vi "Test.vi"() -> ()   [LabVIEW 2021]
uses:
  Commander/Commander.lvclass
  C:/Program Files (x86)/Hyper State Machine Framework/SSW_Hyper_State_Machine.lvlibp/State_Machine_Class/Main_State_Machine/Hyper_State_Machine.lvclass
  Common_State/Common_State.lvclass
  Image_Acquisition/Image_Acquisition.lvclass
  Motion_Control/Motion_Control.lvclass
  Data_Logging/Data_Logging.lvclass
  DIO/DIO.lvclass
  C:/Program Files (x86)/Hyper State Machine Framework/SSW_Hyper_State_Machine.lvlibp/State_Machine_Class/State_Machine_Module.llb/State Machine.ctl
  C:/Program Files (x86)/Hyper State Machine Framework/SSW_Hyper_State_Machine.lvlibp/State_Machine_Class/State_Machine_Module.llb/Lock_Unlock.ctl
  C:/Program Files (x86)/Hyper State Machine Framework/SSW_Hyper_State_Machine.lvlibp/State_Machine_Class/State_Machine_Module.llb/Iterval.ctl
  C:/Program Files (x86)/Hyper State Machine Framework/SSW_Hyper_State_Machine.lvlibp/State_Machine_Class/State_Machine_Module.llb/Time_Out.ctl
  <vilib>/numeric/Random Number (Range) DBL.vi
  <vilib>/Utility/High Resolution Relative Seconds.vi
  C:/Program Files (x86)/Hyper State Machine Framework/SSW_Hyper_State_Machine.lvlibp
panel:
  out "Activate":bool
  out "Lamp":bool
  out "Current_Pos":dbl caption="mm"
  in  "EMO":bool
  out "Product ID":string
  in  "Activate_Code(Blank for 30 min Trial)":string="ROeInPkJ3DxAXwEgzbbW2XA0t1jaS1URlS9jikesQMED6VfU"
  out "Heart_Rate":bool
  out "Heart rate(s)":dbl format="%#_6p"
  out "Execute rate(Hz)":dbl format="%#_6p"
  out "Base Class_Time_Act":bool
  out "Base Class_Elapsed Time(s)":dbl format="%#_6p"
  out "Base Class":bool=TRUE
  out "Base Class_Remaining(s)":dbl format="%#_6p"
  out "Base Class Progress":dbl(slide) scale=0.0..10.0
  in  "Base Class":dbl=10.0 max=1000.0 format="%#_13p"
  out "Base Class":string
  out "Base Class_Active":bool
  in  "Action Manager":T1(ring)
  out "Common":bool=TRUE
  out "Common_State":string
  out "Common_Time_Act":bool
  out "Common_Elapsed Time(s)":dbl format="%#_6p"
  out "Common_State Progress":dbl(slide) scale=0.0..5.0
  in  "Common_State_Interval":dbl=5.0 max=1000.0 format="%#_13p"
  out "Common_State_Active":bool
  out "Common_State_Remaining(s)":dbl format="%#_6p"
  out "Data Logging Progress":dbl(slide) scale=0.0..3.0
  out "DIO Progress":dbl(slide) scale=0.0..0.01
  out "Motion Control Progress":dbl(slide) scale=0.0..0.5
  out "Image Acquisition Progress":dbl(slide) scale=0.0..0.25
  out "Commander Progress":dbl(slide)=-1.0 scale=0.0..1.0
  out "Data_Logging":bool=TRUE
  out "Data Logging":string
  out "Data_Logging_Time_Act":bool
  out "Data_Logging_Elapsed Time(s)":dbl format="%#_6p"
  out "DIO":bool=TRUE
  out "DIO":string
  out "DIO_Time_Act":bool
  out "DIO_Elapsed Time(s)":dbl format="%#_6p"
  out "Motion_Control":bool=TRUE
  out "Motion_Control":string
  out "Motion_Control_Time_Act":bool
  out "Motion_Control_Elapsed Time(s)":dbl format="%#_6p"
  in  "Data Logging":dbl=3.0 max=1000.0 format="%#_13p"
  out "Data Logging_Active":bool
  out "Data Logging_Remaining(s)":dbl format="%#_6p"
  in  "DIO_Interval":dbl=0.01 max=1000.0 format="%#_13p"
  in  "Motion_Control_Interval":dbl=0.5 max=1000.0 format="%#_13p"
  out "Motion Control_Act":bool
  out "DIO_Act":bool
  out "DIO_Remaining(s)":dbl format="%#_6p"
  out "Motion_Control_Remaining(s)":dbl format="%#_6p"
  in  "Image Acquisition_Interval":dbl=0.25 max=1000.0 format="%#_13p"
  in  "Commander_Interval":dbl max=1000.0 format="%#_13p"
  in  "System_Wait_Time":dbl=0.025 format="%#_13p"
  out "Commander_Active":bool
  out "Image Acquisition_Act":bool
  out "Image Acquisition_Remaining(s)":dbl format="%#_6p"
  out "Commander_Remaining(s)":dbl format="%#_6p"
  out "Image Acquisition":bool=TRUE
  out "Image Acquisition":string
  out "Commander":bool=TRUE
  out "Image Acquisition_Time_Act":bool
  out "Image Acquisition_Elapsed Time(s)":dbl format="%#_6p"
  out "Commander":string
  out "State1_Time_Act":bool
  out "Commander_Elapsed Time(s)":dbl format="%#_6p"
  in  "Stop":bool
  # "Note : Each State is Waiting Until Commader State Finished on \"Interval_Delay\" and then Unlock"
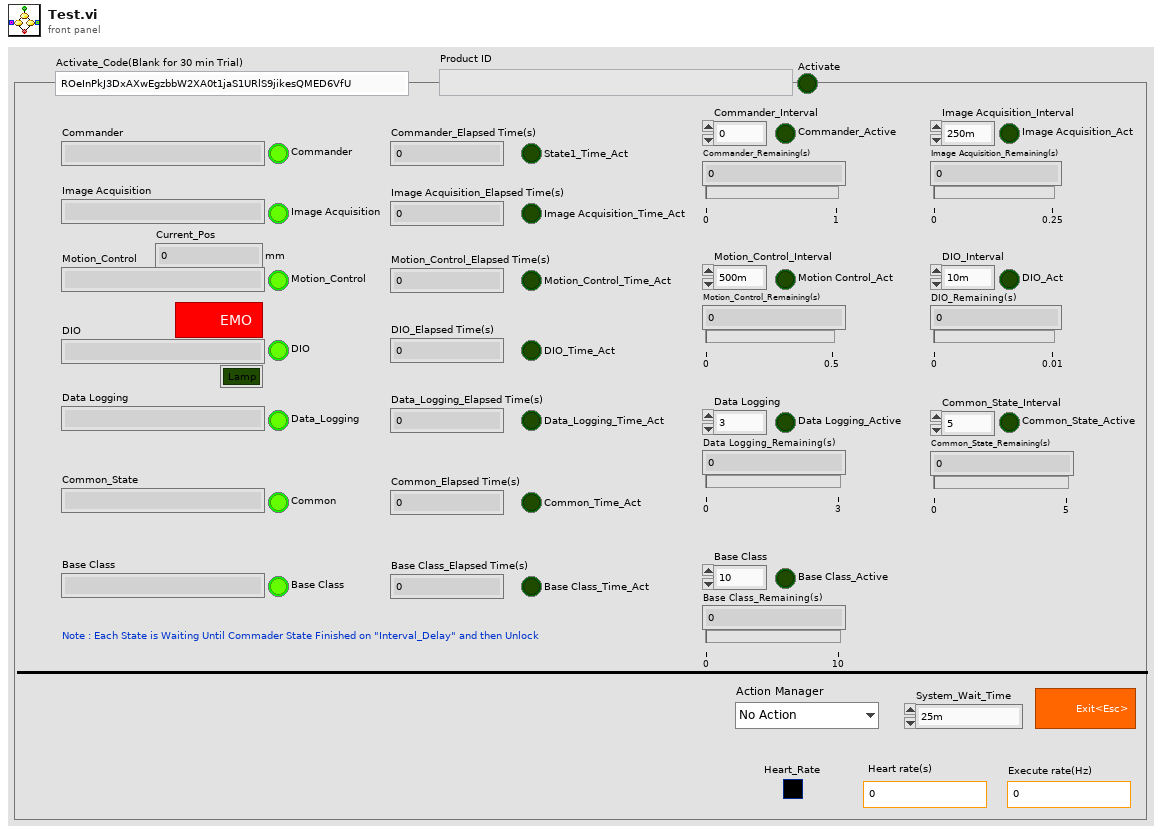
[diagram p1: front panel]
types:
  T1 = enum16{"No Action", "Init", "Lock", "Unlock", "Release"}
  T2 = typedef "SSW_Hyper_State_Machine.lvlibp/State Machine.ctl" = cluster{"Command":string, "Data":variant}
  T3 = typedef "SSW_Hyper_State_Machine.lvlibp/Time_Out.ctl" = cluster{"Enable(True)":bool, "Time Out_State Name":string, "Time Target (1s)":dbl, "Time Out_Reply Message_State":string}
  T4 = typedef "SSW_Hyper_State_Machine.lvlibp/Lock_Unlock.ctl" = cluster{"Action_Mode (Get)":enum16{"Set", "Get"}, "Action_Set (False)":bool, "State_In (Wait)":string}
  T5 = typedef "SSW_Hyper_State_Machine.lvlibp/Iterval.ctl" = cluster{"Delay(s)":dbl, "State (Interval_Delay)":string}
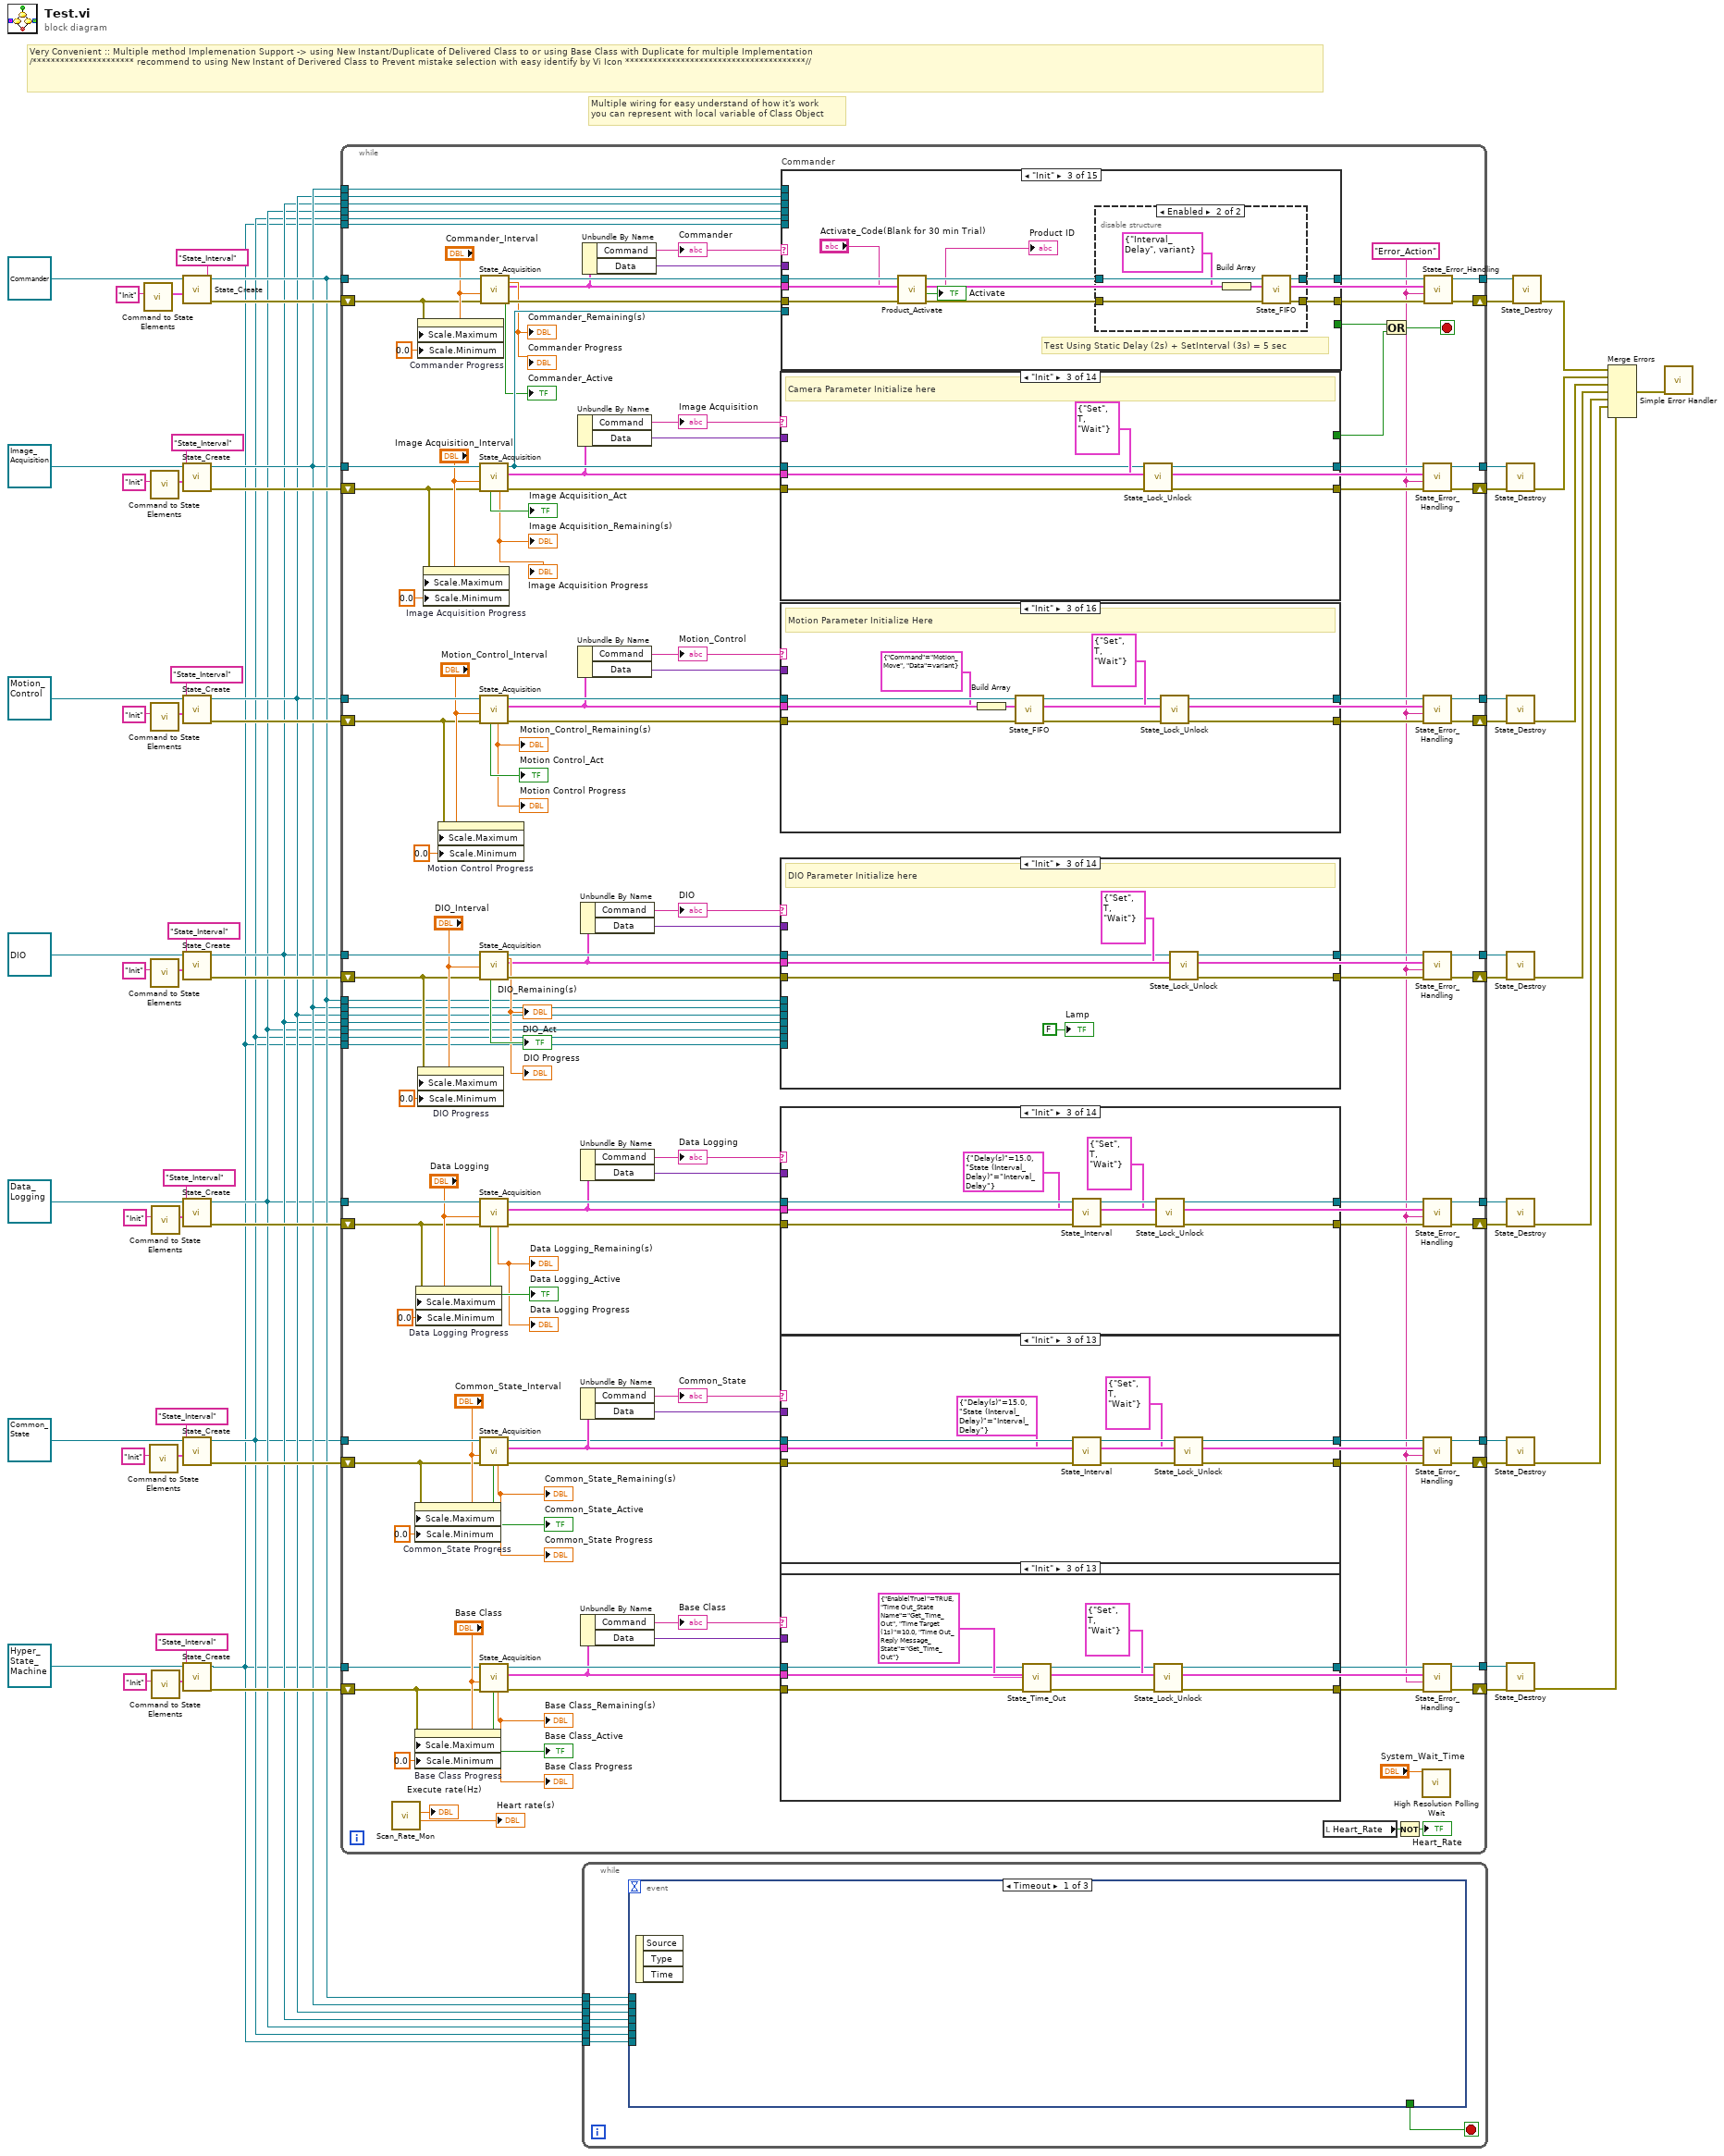
[diagram p0: block diagram]
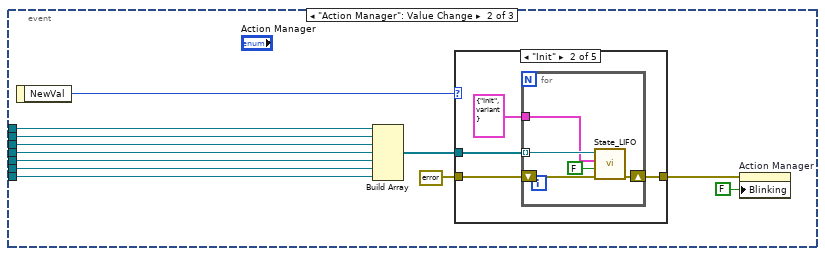
[diagram p2: hidden frame]
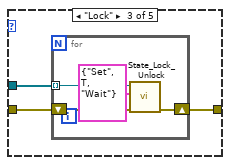
[diagram p4: hidden frame]
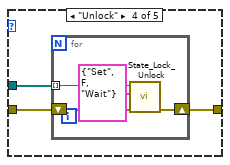
[diagram p5: hidden frame]
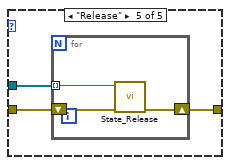
[diagram p6: hidden frame]
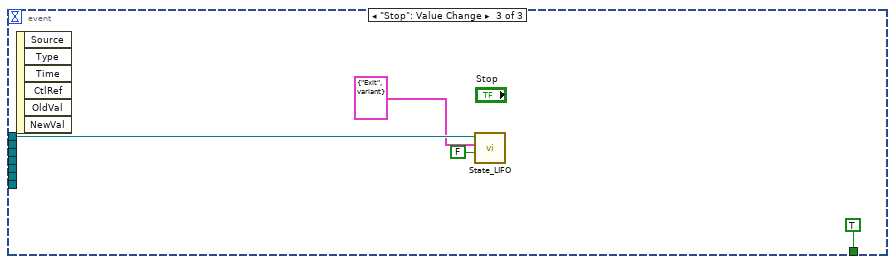
[diagram p7: hidden frame]
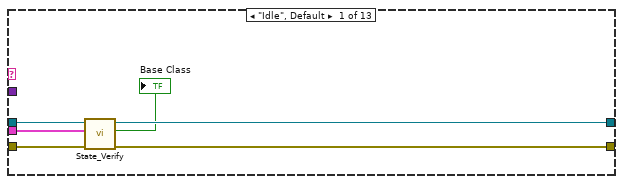
[diagram p8: hidden frame]
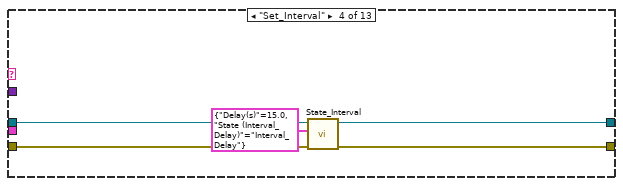
[diagram p10: hidden frame]
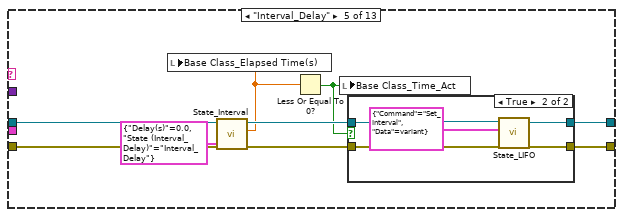
[diagram p11: hidden frame]
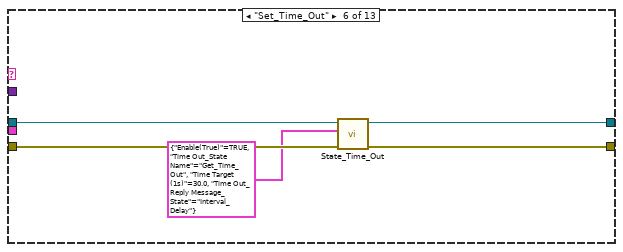
[diagram p13: hidden frame]
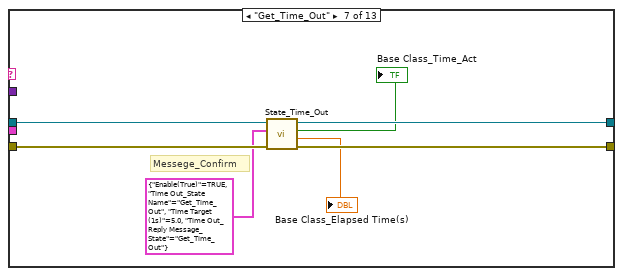
[diagram p14: hidden frame]
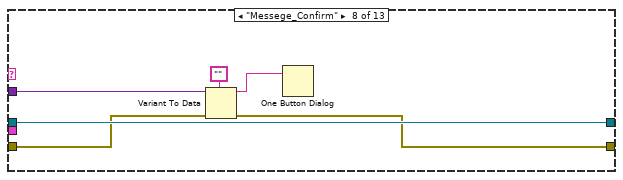
[diagram p15: hidden frame]
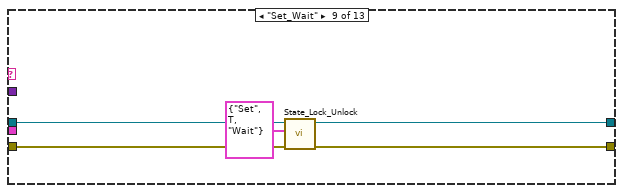
[diagram p16: hidden frame]
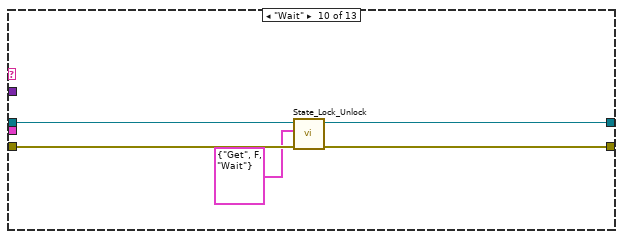
[diagram p17: hidden frame]
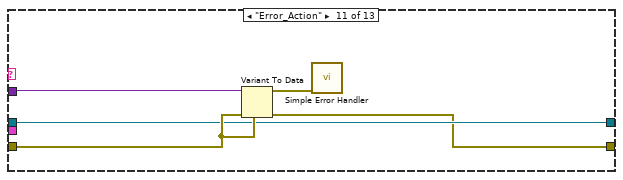
[diagram p18: hidden frame]
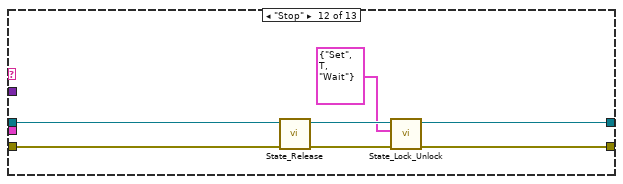
[diagram p19: hidden frame]
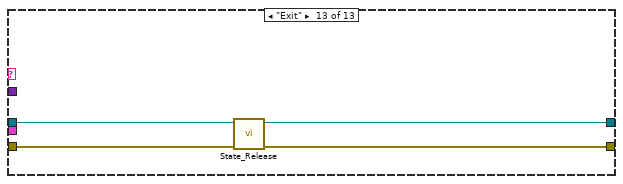
[diagram p20: hidden frame]
diagram:
  # "Multiple wiring for easy understand of how it's work\nyou can represent with local variable of Class Object"
  # "Very Convenient :: Multiple method Implemenation Support -> using New Instant/Duplicate of Delivered Class to or using Base Class with Duplicate for multiple Implementation\n/********************** recommend to using New Instant of Derivered Class to Prevent mistake selection with easy identify by Vi Icon ***************************************//"
  n1 = call "Command to State Elements.vi"("Command"="Init") -> ("Command to State Elements"=w25:T2)  [unwired: 10 in]
  n2 = call "Command to State Elements.vi"("Command"="Init") -> ("Command to State Elements"=w17:T2)  [unwired: 10 in]
  n3 = call "Command to State Elements.vi"("Command"="Init") -> ("Command to State Elements"=w27:T2)  [unwired: 10 in]
  n4 = call "Command to State Elements.vi"("Command"="Init") -> ("Command to State Elements"=w23:T2)  [unwired: 10 in]
  n5 = call "Command to State Elements.vi"("Command"="Init") -> ("Command to State Elements"=w21:T2)  [unwired: 10 in]
  n6 = call "Command to State Elements.vi"("Command"="Init") -> ("Command to State Elements"=w19:T2)  [unwired: 10 in]
  n7 = call "Command to State Elements.vi"("Command"="Init") -> ("Command to State Elements"=w15:T2)  [unwired: 10 in]
  n8 = call-dynamic "State_Create.vi"("Init_State(Option)"=w25, "State_Interval_Name"="State_Interval" ("Core_Interval_Name(State_Interval)"), "State_Machine_Class in"=refnum<class "Commander.lvclass"> refnum ("Commander.lvclass")) -> ("error out"=w64:errorcluster, "State_Machine_Class out"=w7:refnum<class "Commander.lvclass">)  [unwired: 6 in, 1 out]
  n9 = call-dynamic "State_Create.vi"("Init_State(Option)"=w27, "State_Interval_Name"="State_Interval" ("Core_Interval_Name(State_Interval)"), "State_Machine_Class in"=refnum<class "Image_Acquisition.lvclass"> refnum ("Image_Acquisition.lvclass")) -> ("error out"=w61:errorcluster, "State_Machine_Class out"=w6:refnum<class "Image_Acquisition.lvclass">)  [unwired: 6 in, 1 out]
  n10 = call-dynamic "State_Create.vi"("Init_State(Option)"=w23, "State_Interval_Name"="State_Interval" ("Core_Interval_Name(State_Interval)"), "State_Machine_Class in"=refnum<class "Motion_Control.lvclass"> refnum ("Motion_Control.lvclass")) -> ("error out"=w49:errorcluster, "State_Machine_Class out"=w5:refnum<class "Motion_Control.lvclass">)  [unwired: 6 in, 1 out]
  n11 = call-dynamic "State_Create.vi"("Init_State(Option)"=w21, "State_Interval_Name"="State_Interval" ("Core_Interval_Name(State_Interval)"), "State_Machine_Class in"=refnum<class "DIO.lvclass"> refnum ("DIO.lvclass")) -> ("error out"=w47:errorcluster, "State_Machine_Class out"=w4:refnum<class "DIO.lvclass">)  [unwired: 6 in, 1 out]
  n12 = call-dynamic "State_Create.vi"("Init_State(Option)"=w19, "State_Interval_Name"="State_Interval" ("Core_Interval_Name(State_Interval)"), "State_Machine_Class in"=refnum<class "Data_Logging.lvclass"> refnum ("Data_Logging.lvclass")) -> ("error out"=w43:errorcluster, "State_Machine_Class out"=w3:refnum<class "Data_Logging.lvclass">)  [unwired: 6 in, 1 out]
  n13 = call-dynamic "State_Create.vi"("Init_State(Option)"=w17, "State_Interval_Name"="State_Interval" ("Core_Interval_Name(State_Interval)"), "State_Machine_Class in"=refnum<class "Common_State.lvclass"> refnum ("Common_State.lvclass")) -> ("error out"=w38:errorcluster, "State_Machine_Class out"=w2:refnum<class "Common_State.lvclass">)  [unwired: 6 in, 1 out]
  n14 = call-dynamic "State_Create.vi"("Init_State(Option)"=w15, "State_Interval_Name"="State_Interval" ("Core_Interval_Name(State_Interval)"), "State_Machine_Class in"=refnum<class "Hyper_State_Machine.lvclass"> refnum ("SSW_Hyper_State_Machine.lvlibp:Hyper_State_Machine.lvclass")) -> ("error out"=w32:errorcluster, "State_Machine_Class out"=w1:refnum<class "Hyper_State_Machine.lvclass">)  [unwired: 6 in, 1 out]
  n15 = while {
    tunnel: w7 -> [w176]
    shift-right: [w185] -> w63
    shift-left: w64 -> [w84]
    tunnel: [w184] -> w62
    tunnel: w6 -> [w180]
    tunnel: [w179] -> w60
    shift-right: [w178] -> w59
    shift-left: w61 -> [w83]
    tunnel: [w154] -> w51
    tunnel: [w153] -> w50
    tunnel: w5 -> [w152]
    tunnel: w4 -> [w151]
    tunnel: w3 -> [w150]
    shift-right: [w149] -> w48
    shift-left: w49 -> [w82]
    tunnel: [w147] -> w45
    shift-right: [w148] -> w46
    shift-left: w47 -> [w81]
    shift-right: [w146] -> w44
    shift-left: w43 -> [w80]
    tunnel: w2 -> [w125]
    tunnel: [w124] -> w37
    shift-right: [w123] -> w36
    shift-left: w38 -> [w79]
    shift-right: [w93] -> w31
    shift-left: w32 -> [w78]
    tunnel: w1 -> [w97]
    tunnel: [w92] -> w30
    tunnel: w6 -> [w77]
    tunnel: w5 -> [w76]
    tunnel: w4 -> [w75]
    tunnel: w3 -> [w74]
    tunnel: w2 -> [w73]
    tunnel: w1 -> [w72]
    tunnel: w7 -> [w71]
    tunnel: w6 -> [w70]
    tunnel: w5 -> [w69]
    tunnel: w4 -> [w68]
    tunnel: w3 -> [w67]
    tunnel: w2 -> [w66]
    tunnel: w1 -> [w65]
    stop <- w175 stop-if-true
    w91 = "Error_Action" ("State_Error_Handling")
    n16 = call "Scan_Rate_Mon.vi"() -> ("Heart rate(s)"=→"Heart rate(s)":dbl, "Execute rate(Hz)"=→"Execute rate(Hz)":dbl)
    n17 = property on="Common_State Progress" class="Slide (strict)"(error in=w79, "Scale.Maximum"="Common_State_Interval", "Scale.Minimum"=0.0 ("Scale.Range:Minimum")) -> ()  [unwired: 1 in, 2 out]
    n18 = property on="Base Class Progress" class="Slide (strict)"(error in=w78, "Scale.Maximum"="Base Class", "Scale.Minimum"=0.0 ("Scale.Range:Minimum")) -> ()  [unwired: 1 in, 2 out]
    n19 = property on="Data Logging Progress" class="Slide (strict)"(error in=w80, "Scale.Maximum"="Data Logging", "Scale.Minimum"=0.0 ("Scale.Range:Minimum")) -> ()  [unwired: 1 in, 2 out]
    n20 = property on="Commander Progress" class="Slide (strict)"(error in=w84, "Scale.Maximum"="Commander_Interval", "Scale.Minimum"=0.0 ("Scale.Range:Minimum")) -> ()  [unwired: 1 in, 2 out]
    n21 = property on="DIO Progress" class="Slide (strict)"(error in=w81, "Scale.Maximum"="DIO_Interval", "Scale.Minimum"=0.0 ("Scale.Range:Minimum")) -> ()  [unwired: 1 in, 2 out]
    n22 = property on="Image Acquisition Progress" class="Slide (strict)"(error in=w83, "Scale.Maximum"="Image Acquisition_Interval", "Scale.Minimum"=0.0 ("Scale.Range:Minimum")) -> ()  [unwired: 1 in, 2 out]
    n23 = property on="Motion Control Progress" class="Slide (strict)"(error in=w82, "Scale.Maximum"="Motion_Control_Interval", "Scale.Minimum"=0.0 ("Scale.Range:Minimum")) -> ()  [unwired: 1 in, 2 out]
    n24 = call-dynamic "State_Acquisition.vi"("error in (no error)"=w83, "State_Interval_Time(s)"="Image Acquisition_Interval", "Main_Machine_State_Class in"=w180) -> ("error out"=w183:errorcluster, "State"=w110:T2, "Main_Machine_State_Class out"=w177:refnum<class "Image_Acquisition.lvclass">, "Remaining(ms)"=→"Image Acquisition_Remaining(s)" →"Image Acquisition Progress":dbl, "Current_State_Active"=→"Image Acquisition_Act":bool)  [unwired: 2 in, 2 out]
    n25 = call-dynamic "State_Acquisition.vi"("error in (no error)"=w82, "State_Interval_Time(s)"="Motion_Control_Interval", "Main_Machine_State_Class in"=w152) -> ("error out"=w156:errorcluster, "State"=w109:T2, "Main_Machine_State_Class out"=w157:refnum<class "Motion_Control.lvclass">, "Remaining(ms)"=→"Motion_Control_Remaining(s)" →"Motion Control Progress":dbl, "Current_State_Active"=→"Motion Control_Act":bool)  [unwired: 2 in, 2 out]
    n26 = call-dynamic "State_Acquisition.vi"("error in (no error)"=w81, "State_Interval_Time(s)"="DIO_Interval", "Main_Machine_State_Class in"=w151) -> ("error out"=w163:errorcluster, "State"=w108:T2, "Main_Machine_State_Class out"=w164:refnum<class "DIO.lvclass">, "Remaining(ms)"=→"DIO_Remaining(s)" →"DIO Progress":dbl, "Current_State_Active"=→"DIO_Act":bool)  [unwired: 2 in, 2 out]
    n27 = call-dynamic "State_Acquisition.vi"("error in (no error)"=w80, "State_Interval_Time(s)"="Data Logging", "Main_Machine_State_Class in"=w150) -> ("error out"=w165:errorcluster, "State"=w107:T2, "Main_Machine_State_Class out"=w166:refnum<class "Data_Logging.lvclass">, "Remaining(ms)"=→"Data Logging_Remaining(s)" →"Data Logging Progress":dbl, "Current_State_Active"=→"Data Logging_Active":bool)  [unwired: 2 in, 2 out]
    n28 = call-dynamic "State_Acquisition.vi"("error in (no error)"=w79, "State_Interval_Time(s)"="Common_State_Interval", "Main_Machine_State_Class in"=w125) -> ("error out"=w127:errorcluster, "State"=w106:T2, "Main_Machine_State_Class out"=w90:refnum<class "Common_State.lvclass">, "Remaining(ms)"=→"Common_State_Remaining(s)" →"Common_State Progress":dbl, "Current_State_Active"=→"Common_State_Active":bool)  [unwired: 2 in, 2 out]
    n29 = call-dynamic "State_Acquisition.vi"("error in (no error)"=w78, "State_Interval_Time(s)"="Base Class", "Main_Machine_State_Class in"=w97) -> ("error out"=w98:errorcluster, "State"=w95:T2, "Main_Machine_State_Class out"=w99:refnum<class "Hyper_State_Machine.lvclass">, "Remaining(ms)"=→"Base Class_Remaining(s)" →"Base Class Progress":dbl, "Current_State_Active"=→"Base Class_Active":bool)  [unwired: 2 in, 2 out]
    n30 = call-dynamic "State_Acquisition.vi"("error in (no error)"=w84, "State_Interval_Time(s)"="Commander_Interval", "Main_Machine_State_Class in"=w176) -> ("error out"=w187:errorcluster, "State"=w111:T2, "Main_Machine_State_Class out"=w188:refnum<class "Commander.lvclass">, "Remaining(ms)"=→"Commander_Remaining(s)" →"Commander Progress":dbl, "Current_State_Active"=→"Commander_Active":bool)  [unwired: 2 in, 2 out]
    n31 = Unbundle By Name(w110) -> ("Command"=w181:string, "Data"=w182:variant)
    "Image Acquisition" <- w181
    n32 = Unbundle By Name(w109) -> ("Command"=w140:string, "Data"=w169:variant)
    "Motion_Control" <- w140
    n33 = Unbundle By Name(w108) -> ("Command"=w141:string, "Data"=w168:variant)
    "DIO" <- w141
    n34 = Unbundle By Name(w107) -> ("Command"=w142:string, "Data"=w167:variant)
    "Data Logging" <- w142
    n35 = Unbundle By Name(w106) -> ("Command"=w120:string, "Data"=w126:variant)
    "Common_State" <- w120
    n36 = Unbundle By Name(w95) -> ("Command"=w103:string, "Data"=w100:variant)
    "Base Class" <- w103
    n37 = Unbundle By Name(w111) -> ("Command"=w191:string, "Data"=w190:variant)
    "Commander" <- w191
    n38 = case shown="\"Init\"" w181 {
      selector: w181 -> [_ _ _ w666 _ _ _ _ _ _ _ _ _ _]
      tunnel: w182 -> [_ _ _ _ _ _ _ _ w720 _ _ w734 _ _]
      tunnel: w177 -> [w657 w659 w661 w671 w676 w689 w707 w714 w718 w725 w730 w731 w742 w747]
      tunnel: w183 -> [w656 w658 w660 w670 w675 w688 w706 w713 w717 w724 w729 w733 w741 w746]
      tunnel: [w650 w659 w664 w669 w674 w684 w705 w712 w718 w723 w728 w731 w737 w745] -> w171
      tunnel: [w649 w658 w663 w668 w673 w683 w704 w711 w716 w722 w727 w732 w736 w744] -> w170
      tunnel: w110 -> [w655 _ _ _ _ _ _ _ _ _ _ _ _ _]
      tunnel: [_ _ _ _ _ _ _ _ _ _ _ _ _ TRUE] -> w174
      frame "Idle", Default {
        n39 = call-dynamic "State_Verify.vi"("error in (no error)"=w656, "State(Idle)"=w655, "State_Machine_Class in"=w657) -> ("error out"=w652:errorcluster, "Active"=→"Image Acquisition":bool, "State_Machine_Class out"=w653:refnum<class "Image_Acquisition.lvclass">)  [unwired: 6 in]
        n40 = Build Array(T2 {"Command"="Image_Acquisition", "Data"=variant} ("State")) -> (w648:T2[])
        n41 = call-dynamic "State_FIFO.vi"("error in (no error)"=w652, "State Machine[]"=w648, "State_Machine_Class in"=w653) -> ("error out"=w649:errorcluster, "State_Machine_Class out"=w650:refnum<class "Image_Acquisition.lvclass">)  [unwired: 7 in]
      }
      frame "State_Interval" {
      }
      frame "Init" {
        # "Camera Parameter Initialize here"
        n42 = call-dynamic "State_Lock_Unlock.vi"("error in (no error)"=w660, "Parameter"=T4 {"Action_Mode (Get)"=enum."Set", "Action_Set (False)"=TRUE, "State_In (Wait)"="Wait"}, "State_Machine_Class in"=w661) -> ("error out"=w663:errorcluster, "State_Machine_Class out"=w664:refnum<class "Image_Acquisition.lvclass">)  [unwired: 6 in, 1 out]
      }
      frame "Image_Acquisition" {
        (unwired) T5 {"Delay(s)"=5.0, "State (Interval_Delay)"="Image_Acquisition"} ("Parameter")
        # "Simple handling with specify name"
        # "Dynamic handling Name for Waiting Demo"
        # "Image Acquisition Function Here"
        n43 = Bundle By Name(cluster=T5 {"Delay(s)"=5.0, "State (Interval_Delay)"=""} ("Parameter"), "State (Interval_Delay)"=w666) -> (w665:T5)
        n44 = call-dynamic "State_Interval.vi"("error in (no error)"=w670, "Parameter"=w665, "State_Machine_Class in"=w671) -> ("error out"=w668:errorcluster, "State_Machine_Class out"=w669:refnum<class "Image_Acquisition.lvclass">)  [unwired: 6 in, 1 out]
      }
      frame "Set_Interval" {
        n45 = call-dynamic "State_Interval.vi"("error in (no error)"=w675, "Parameter"=T5 {"Delay(s)"=15.0, "State (Interval_Delay)"="Interval_Delay"}, "State_Machine_Class in"=w676) -> ("error out"=w673:errorcluster, "State_Machine_Class out"=w674:refnum<class "Image_Acquisition.lvclass">)  [unwired: 6 in, 1 out]
      }
      frame "Interval_Delay" {
        n46 = call-dynamic "State_Interval.vi"("error in (no error)"=w688, "Parameter"=T5 {"Delay(s)"=0.0, "State (Interval_Delay)"="Interval_Delay"}, "State_Machine_Class in"=w689) -> ("error out"=w685:errorcluster, "Elapsed Time(s)"=w682:dbl, "State_Machine_Class out"=w686:refnum<class "Image_Acquisition.lvclass">)  [unwired: 6 in]
        "Image Acquisition_Elapsed Time(s)" <- w682
        n47 = Build Array(T2 {"Command"="Interval_Delay", "Data"=variant} ("State"), T2 {"Command"="Image_Acquisition", "Data"=variant} ("State")) -> (w678:T2[])
        n48 = Less Or Equal To 0?(x=w682) -> (x <= 0?=w687:bool)
        n49 = Reverse 1D Array(array=w678) -> (reversed array=w677:T2[])
        n50 = case shown="True" w687 {
          tunnel: w686 -> [w691 w696]
          tunnel: w685 -> [w690 w695]
          tunnel: [w691 w694] -> w684
          tunnel: [w690 w693] -> w683
          tunnel: w677 -> [_ w692]
          frame False {
          }
          frame True {
            n51 = for {
              shift-right: [w699] -> w694
              shift-left: w696 -> [w701]
              shift-right: [w698] -> w693
              shift-left: w695 -> [w700]
              tunnel: w692 -> [w697] mode=indexing
              n52 = call-dynamic "State_LIFO.vi"("error in (no error)"=w700, "State Machine"=w697, "State_Machine_Class in"=w701) -> ("error out"=w698:errorcluster, "State_Machine_Class out"=w699:refnum<class "Image_Acquisition.lvclass">)  [unwired: 7 in]
            }
          }
        }
        n53 = local write "Image Acquisition_Time_Act"(w687) -> ()
      }
      frame "Set_Time_Out" {
        n54 = call-dynamic "State_Time_Out.vi"("error in (no error)"=w706, "Parameter"=T3 {"Enable(True)"=TRUE, "Time Out_State Name"="Get_Time_Out", "Time Target (1s)"=30.0, "Time Out_Reply Message_State"="Messege_Confirm"}, "State_Machine_Class in"=w707) -> ("error out"=w704:errorcluster, "Timeout"=w703:bool, "State_Machine_Class out"=w705:refnum<class "Image_Acquisition.lvclass">)  [unwired: 5 in, 1 out]
        n55 = local write "Image Acquisition_Time_Act"(w703) -> ()
      }
      frame "Get_Time_Out" {
        # "Messege_Confirm"
        n56 = call-dynamic "State_Time_Out.vi"("error in (no error)"=w713, "Parameter"=T3 {"Enable(True)"=TRUE, "Time Out_State Name"="Get_Time_Out", "Time Target (1s)"=0.0, "Time Out_Reply Message_State"="Messege_Confirm"}, "State_Machine_Class in"=w714) -> ("error out"=w711:errorcluster, "Remaining Time (s)"=w710:dbl, "Timeout"=→"Image Acquisition_Time_Act":bool, "State_Machine_Class out"=w712:refnum<class "Image_Acquisition.lvclass">)  [unwired: 5 in]
        n57 = local write "Image Acquisition_Elapsed Time(s)"(w710) -> ()
      }
      frame "Messege_Confirm" {
        n58 = Variant To Data(error in=w717, type="", Variant=w720) -> (data=w715:string, error out=w716:errorcluster)
        n59 = One Button Dialog(message=w715) -> ()  [unwired: 1 in, 1 out]
      }
      frame "Set_Wait" {
        n60 = call-dynamic "State_Lock_Unlock.vi"("error in (no error)"=w724, "Parameter"=T4 {"Action_Mode (Get)"=enum."Set", "Action_Set (False)"=TRUE, "State_In (Wait)"="Wait"}, "State_Machine_Class in"=w725) -> ("error out"=w722:errorcluster, "State_Machine_Class out"=w723:refnum<class "Image_Acquisition.lvclass">)  [unwired: 6 in, 1 out]
      }
      frame "Wait" {
        n61 = call-dynamic "State_Lock_Unlock.vi"("error in (no error)"=w729, "Parameter"=T4 {"Action_Mode (Get)"=enum."Get", "Action_Set (False)"=FALSE, "State_In (Wait)"="Wait"}, "State_Machine_Class in"=w730) -> ("error out"=w727:errorcluster, "State_Machine_Class out"=w728:refnum<class "Image_Acquisition.lvclass">)  [unwired: 6 in, 1 out]
      }
      frame "Error_Action" {
        n62 = Variant To Data(error in=w733, type=w733, Variant=w734) -> (data=w735:errorcluster, error out=w732:errorcluster)
        n63 = call <vilib>:"Simple Error Handler.vi"("error in (no error)"=w735) -> ()  [unwired: 4 in, 5 out]
      }
      frame "Stop" {
        n64 = call-dynamic "State_Release.vi"("error in (no error)"=w741, "State_Machine_Class in"=w742) -> ("error out"=w739:errorcluster, "State_Machine_Class out"=w740:refnum<class "Image_Acquisition.lvclass">)  [unwired: 8 in]
        n65 = call-dynamic "State_Lock_Unlock.vi"("error in (no error)"=w739, "Parameter"=T4 {"Action_Mode (Get)"=enum."Set", "Action_Set (False)"=TRUE, "State_In (Wait)"="Wait"}, "State_Machine_Class in"=w740) -> ("error out"=w736:errorcluster, "State_Machine_Class out"=w737:refnum<class "Image_Acquisition.lvclass">)  [unwired: 6 in, 1 out]
      }
      frame "Exit" {
        n66 = call-dynamic "State_Release.vi"("error in (no error)"=w746, "State_Machine_Class in"=w747) -> ("error out"=w744:errorcluster, "State_Machine_Class out"=w745:refnum<class "Image_Acquisition.lvclass">)  [unwired: 8 in]
      }
    }
    n67 = case shown="\"Init\"" w140 {
      tunnel: w169 -> [_ _ _ _ _ _ _ _ _ _ w621 _ _ w634 _ _]
      tunnel: w157 -> [w557 w559 w565 w573 w578 w581 w586 w595 w608 w615 w619 w626 w631 w635 w643 w647]
      tunnel: w156 -> [w556 w558 w563 w572 w577 w580 w585 w594 w607 w614 w618 w625 w630 w633 w642 w646]
      tunnel: [w550 w559 w567 w571 w576 w581 w584 w591 w606 w613 w619 w624 w629 w635 w639 w645] -> w158
      tunnel: [w549 w558 w566 w570 w575 w580 w583 w590 w605 w612 w617 w623 w628 w632 w638 w644] -> w155
      tunnel: w109 -> [w555 _ _ _ _ _ _ _ _ _ _ _ _ _ _ _]
      frame "Idle", Default {
        n68 = call-dynamic "State_Verify.vi"("error in (no error)"=w556, "State(Idle)"=w555, "State_Machine_Class in"=w557) -> ("error out"=w552:errorcluster, "Active"=→"Motion_Control":bool, "State_Machine_Class out"=w553:refnum<class "Motion_Control.lvclass">)  [unwired: 6 in]
        n69 = Build Array(T2 {"Command"="Motion_Move", "Data"=variant} ("State")) -> (w548:T2[])
        n70 = call-dynamic "State_FIFO.vi"("error in (no error)"=w552, "State Machine[]"=w548, "State_Machine_Class in"=w553) -> ("error out"=w549:errorcluster, "State_Machine_Class out"=w550:refnum<class "Motion_Control.lvclass">)  [unwired: 7 in]
      }
      frame "State_Interval" {
        # "Handling Motion I/O or Cirtical Task Here"
      }
      frame "Init" {
        # "Motion Parameter Initialize Here"
        n71 = Build Array(T2 {"Command"="Motion_Move", "Data"=variant} ("State")) -> (w560:T2[])
        n72 = call-dynamic "State_FIFO.vi"("error in (no error)"=w563, "State Machine[]"=w560, "State_Machine_Class in"=w565) -> ("error out"=w562:errorcluster, "State_Machine_Class out"=w564:refnum<class "Motion_Control.lvclass">)  [unwired: 7 in]
        n73 = call-dynamic "State_Lock_Unlock.vi"("error in (no error)"=w562, "Parameter"=T4 {"Action_Mode (Get)"=enum."Set", "Action_Set (False)"=TRUE, "State_In (Wait)"="Wait"}, "State_Machine_Class in"=w564) -> ("error out"=w566:errorcluster, "State_Machine_Class out"=w567:refnum<class "Motion_Control.lvclass">)  [unwired: 6 in, 1 out]
      }
      frame "Motion_Move" {
        # "Motion Move Command here"
        n74 = call-dynamic "State_LIFO.vi"("error in (no error)"=w572, "State Machine"=T2 {"Command"="Motion_Request_Pos", "Data"=variant} ("State"), "State_Machine_Class in"=w573) -> ("error out"=w570:errorcluster, "State_Machine_Class out"=w571:refnum<class "Motion_Control.lvclass">)  [unwired: 7 in]
      }
      frame "Motion_Request_Pos" {
        # "Motion Query Position Command here"
        n75 = call-dynamic "State_LIFO.vi"("error in (no error)"=w577, "State Machine"=T2 {"Command"="Motion_Get_Pos", "Data"=variant} ("State"), "State_Machine_Class in"=w578) -> ("error out"=w575:errorcluster, "State_Machine_Class out"=w576:refnum<class "Motion_Control.lvclass">)  [unwired: 7 in]
      }
      frame "Motion_Get_Pos" {
        # "Motion Move Command here"
        n76 = call-poly <vilib>:"Random Number (Range).vi"() -> ("number"=→"Current_Pos":dbl)  [unwired: 11 in]
      }
      frame "Set_Interval" {
        n77 = call-dynamic "State_Interval.vi"("error in (no error)"=w585, "Parameter"=T5 {"Delay(s)"=15.0, "State (Interval_Delay)"="Interval_Delay"}, "State_Machine_Class in"=w586) -> ("error out"=w583:errorcluster, "State_Machine_Class out"=w584:refnum<class "Motion_Control.lvclass">)  [unwired: 6 in, 1 out]
      }
      frame "Interval_Delay" {
        n78 = call-dynamic "State_Interval.vi"("error in (no error)"=w594, "Parameter"=T5 {"Delay(s)"=0.0, "State (Interval_Delay)"="Interval_Delay"}, "State_Machine_Class in"=w595) -> ("error out"=w592:errorcluster, "Elapsed Time(s)"=w589:dbl, "State_Machine_Class out"=w593:refnum<class "Motion_Control.lvclass">)  [unwired: 6 in]
        n79 = local write "Motion_Control_Elapsed Time(s)"(w589) -> ()
        n80 = Less Or Equal To 0?(x=w589) -> (x <= 0?=w588:bool)
        n81 = local write "Motion_Control_Time_Act"(w588) -> ()
        n82 = case shown="True" w588 {
          tunnel: w593 -> [w597 w603]
          tunnel: w592 -> [w596 w602]
          tunnel: [w597 w601] -> w591
          tunnel: [w596 w600] -> w590
          frame False {
          }
          frame True {
            n83 = call-dynamic "State_LIFO.vi"("error in (no error)"=w602, "State_Interval(Enable)"=FALSE, "State Machine"=T2 {"Command"="Set_Interval", "Data"=variant} ("State"), "State_Machine_Class in"=w603) -> ("error out"=w600:errorcluster, "State_Machine_Class out"=w601:refnum<class "Motion_Control.lvclass">)  [unwired: 6 in]
          }
        }
      }
      frame "Set_Time_Out" {
        n84 = call-dynamic "State_Time_Out.vi"("error in (no error)"=w607, "Parameter"=T3 {"Enable(True)"=TRUE, "Time Out_State Name"="Get_Time_Out", "Time Target (1s)"=30.0, "Time Out_Reply Message_State"="Messege_Confirm"}, "State_Machine_Class in"=w608) -> ("error out"=w605:errorcluster, "State_Machine_Class out"=w606:refnum<class "Motion_Control.lvclass">)  [unwired: 5 in, 2 out]
      }
      frame "Get_Time_Out" {
        # "Messege_Confirm"
        n85 = call-dynamic "State_Time_Out.vi"("error in (no error)"=w614, "Parameter"=T3 {"Enable(True)"=TRUE, "Time Out_State Name"="Get_Time_Out", "Time Target (1s)"=0.0, "Time Out_Reply Message_State"="Messege_Confirm"}, "State_Machine_Class in"=w615) -> ("error out"=w612:errorcluster, "Remaining Time (s)"=→"Motion_Control_Elapsed Time(s)":dbl, "Timeout"=→"Motion_Control_Time_Act":bool, "State_Machine_Class out"=w613:refnum<class "Motion_Control.lvclass">)  [unwired: 5 in]
      }
      frame "Messege_Confirm" {
        n86 = Variant To Data(error in=w618, type="", Variant=w621) -> (data=w616:string, error out=w617:errorcluster)
        n87 = One Button Dialog(message=w616) -> ()  [unwired: 1 in, 1 out]
      }
      frame "Set_Wait" {
        n88 = call-dynamic "State_Lock_Unlock.vi"("error in (no error)"=w625, "Parameter"=T4 {"Action_Mode (Get)"=enum."Set", "Action_Set (False)"=TRUE, "State_In (Wait)"="Wait"}, "State_Machine_Class in"=w626) -> ("error out"=w623:errorcluster, "State_Machine_Class out"=w624:refnum<class "Motion_Control.lvclass">)  [unwired: 6 in, 1 out]
      }
      frame "Wait" {
        n89 = call-dynamic "State_Lock_Unlock.vi"("error in (no error)"=w630, "Parameter"=T4 {"Action_Mode (Get)"=enum."Get", "Action_Set (False)"=FALSE, "State_In (Wait)"="Wait"}, "State_Machine_Class in"=w631) -> ("error out"=w628:errorcluster, "State_Machine_Class out"=w629:refnum<class "Motion_Control.lvclass">)  [unwired: 6 in, 1 out]
      }
      frame "Error_Action" {
        n90 = Variant To Data(error in=w633, type=w633, Variant=w634) -> (data=w636:errorcluster, error out=w632:errorcluster)
        n91 = call <vilib>:"Simple Error Handler.vi"("error in (no error)"=w636) -> ()  [unwired: 4 in, 5 out]
      }
      frame "Stop" {
        n92 = call-dynamic "State_Release.vi"("error in (no error)"=w642, "State_Machine_Class in"=w643) -> ("error out"=w640:errorcluster, "State_Machine_Class out"=w641:refnum<class "Motion_Control.lvclass">)  [unwired: 8 in]
        n93 = call-dynamic "State_Lock_Unlock.vi"("error in (no error)"=w640, "Parameter"=T4 {"Action_Mode (Get)"=enum."Set", "Action_Set (False)"=TRUE, "State_In (Wait)"="Wait"}, "State_Machine_Class in"=w641) -> ("error out"=w638:errorcluster, "State_Machine_Class out"=w639:refnum<class "Motion_Control.lvclass">)  [unwired: 6 in, 1 out]
      }
      frame "Exit" {
        n94 = call-dynamic "State_Release.vi"("error in (no error)"=w646, "State_Machine_Class in"=w647) -> ("error out"=w644:errorcluster, "State_Machine_Class out"=w645:refnum<class "Motion_Control.lvclass">)  [unwired: 8 in]
      }
    }
    n95 = case shown="\"Init\"" w141 {
      tunnel: w168 -> [_ _ _ _ _ _ _ _ w518 _ _ w531 _ _]
      tunnel: w164 -> [w448 w458 w475 w484 w491 w496 w503 w509 w516 w523 w528 w529 w543 w547]
      tunnel: w163 -> [w447 w449 w474 w483 w490 w495 w502 w508 w515 w522 w527 w532 w542 w546]
      tunnel: [w442 w458 w479 w482 w486 w494 w501 w507 w516 w521 w526 w529 w539 w545] -> w162
      tunnel: [w441 w449 w478 w481 w485 w493 w500 w506 w514 w520 w525 w530 w536 w544] -> w161
      tunnel: w108 -> [w446 _ _ _ _ _ _ _ _ _ _ _ _ _]
      tunnel: w71 -> [_ w456 _ _ _ _ _ _ _ _ _ _ _ _]
      tunnel: w70 -> [_ w455 _ _ _ _ _ _ _ _ _ _ _ _]
      tunnel: w69 -> [_ w454 _ _ _ _ _ _ _ _ _ _ _ _]
      tunnel: w68 -> [_ w453 _ _ _ _ _ _ _ _ _ _ _ _]
      tunnel: w67 -> [_ w452 _ _ _ _ _ _ _ _ _ _ _ _]
      tunnel: w66 -> [_ w451 _ _ _ _ _ _ _ _ _ _ _ _]
      tunnel: w65 -> [_ w450 _ _ _ _ _ _ _ _ _ _ _ _]
      frame "Idle", Default {
        # "Able to activate at \"Stae_Interval\""
        n96 = call-dynamic "State_Verify.vi"("error in (no error)"=w447, "State(Idle)"=w446, "State_Machine_Class in"=w448) -> ("error out"=w443:errorcluster, "Active"=→"DIO":bool, "State_Machine_Class out"=w444:refnum<class "DIO.lvclass">)  [unwired: 6 in]
        n97 = Build Array(T2 {"Command"="Lamp_Blinking", "Data"=variant} ("State")) -> (w439:T2[])
        n98 = call-dynamic "State_FIFO.vi"("error in (no error)"=w443, "State Machine[]"=w439, "State_Machine_Class in"=w444) -> ("error out"=w441:errorcluster, "State_Machine_Class out"=w442:refnum<class "DIO.lvclass">)  [unwired: 7 in]
      }
      frame "State_Interval" {
        # "Able to assign to Even to handling"
        # "Simulation of Emergency Signal , Pree to try (Can not Override State Lock if in Active)"
        # "Simulation of Emergency Signal"
        # "Every Cycle Time DIO Get Data Here"
        n99 = case shown="True" "EMO" {
          tunnel: w456 -> [_ w468]
          tunnel: w455 -> [_ w467]
          tunnel: w454 -> [_ w466]
          tunnel: w453 -> [_ w465]
          tunnel: w452 -> [_ w464]
          tunnel: w451 -> [_ w463]
          tunnel: w450 -> [_ w462]
          tunnel: w449 -> [_ w459]
          frame False {
          }
          frame True {
            n100 = Build Array(w468, w467, w466, w465, w464, w463, w462) -> (w461:refnum<class "Hyper_State_Machine.lvclass">[])
            n101 = for {
              tunnel: w461 -> [w473] mode=indexing
              tunnel: T2 {"Command"="Stop", "Data"=variant} ("State") -> [w469]
              shift-right: [w471] -> _
              shift-left: w459 -> [w472]
              n102 = call-dynamic "State_LIFO.vi"("error in (no error)"=w472, "State_Interval(Enable)"=FALSE, "State Machine"=w469, "State_Machine_Class in"=w473) -> ("error out"=w471:errorcluster)  [unwired: 6 in, 1 out]
            }
          }
        }
      }
      frame "Init" {
        # "DIO Parameter Initialize here"
        n103 = call-dynamic "State_Lock_Unlock.vi"("error in (no error)"=w474, "Parameter"=T4 {"Action_Mode (Get)"=enum."Set", "Action_Set (False)"=TRUE, "State_In (Wait)"="Wait"}, "State_Machine_Class in"=w475) -> ("error out"=w478:errorcluster, "State_Machine_Class out"=w479:refnum<class "DIO.lvclass">)  [unwired: 6 in, 1 out]
        "Lamp" <- FALSE ("Lamp")
      }
      frame "Set_Interval" {
        n104 = call-dynamic "State_Interval.vi"("error in (no error)"=w483, "Parameter"=T5 {"Delay(s)"=15.0, "State (Interval_Delay)"="Interval_Delay"}, "State_Machine_Class in"=w484) -> ("error out"=w481:errorcluster, "State_Machine_Class out"=w482:refnum<class "DIO.lvclass">)  [unwired: 6 in, 1 out]
      }
      frame "Interval_Delay" {
        n105 = call-dynamic "State_Interval.vi"("error in (no error)"=w490, "Parameter"=T5 {"Delay(s)"=0.0, "State (Interval_Delay)"="Interval_Delay"}, "State_Machine_Class in"=w491) -> ("error out"=w485:errorcluster, "Elapsed Time(s)"=w489:dbl, "State_Machine_Class out"=w486:refnum<class "DIO.lvclass">)  [unwired: 6 in]
        n106 = local write "DIO_Elapsed Time(s)"(w489) -> ()
        n107 = Less Or Equal To 0?(x=w489) -> (x <= 0?=w488:bool)
        n108 = local write "DIO_Time_Act"(w488) -> ()
      }
      frame "Set_Time_Out" {
        n109 = call-dynamic "State_Time_Out.vi"("error in (no error)"=w495, "Parameter"=T3 {"Enable(True)"=TRUE, "Time Out_State Name"="Get_Time_Out", "Time Target (1s)"=30.0, "Time Out_Reply Message_State"="Messege_Confirm"}, "State_Machine_Class in"=w496) -> ("error out"=w493:errorcluster, "State_Machine_Class out"=w494:refnum<class "DIO.lvclass">)  [unwired: 5 in, 2 out]
      }
      frame "Get_Time_Out" {
        # "Messege_Confirm"
        n110 = call-dynamic "State_Time_Out.vi"("error in (no error)"=w502, "Parameter"=T3 {"Enable(True)"=TRUE, "Time Out_State Name"="Get_Time_Out", "Time Target (1s)"=0.0, "Time Out_Reply Message_State"="Messege_Confirm"}, "State_Machine_Class in"=w503) -> ("error out"=w500:errorcluster, "Remaining Time (s)"=→"DIO_Elapsed Time(s)":dbl, "Timeout"=→"DIO_Time_Act":bool, "State_Machine_Class out"=w501:refnum<class "DIO.lvclass">)  [unwired: 5 in]
      }
      frame "Lamp_Blinking" {
        n111 = call-dynamic "State_Interval.vi"("error in (no error)"=w508, "Parameter"=T5 {"Delay(s)"=0.25, "State (Interval_Delay)"="Lamp_Blinking"}, "State_Machine_Class in"=w509) -> ("error out"=w506:errorcluster, "Elapsed Time(s)"=w504:dbl, "State_Machine_Class out"=w507:refnum<class "DIO.lvclass">)  [unwired: 6 in]
        n112 = Less Or Equal To 0?(x=w504) -> (x <= 0?=w505:bool)
        n113 = case shown="True" w505 {
          frame False {
          }
          frame True {
            n114 = local read "Lamp"() -> (w512:bool)
            n115 = Not(x=w512) -> (.not. x?=w511:bool)
            n116 = local write "Lamp"(w511) -> ()
          }
        }
      }
      frame "Messege_Confirm" {
        n117 = Variant To Data(error in=w515, type="", Variant=w518) -> (data=w513:string, error out=w514:errorcluster)
        n118 = One Button Dialog(message=w513) -> ()  [unwired: 1 in, 1 out]
      }
      frame "Set_Wait" {
        n119 = call-dynamic "State_Lock_Unlock.vi"("error in (no error)"=w522, "Parameter"=T4 {"Action_Mode (Get)"=enum."Set", "Action_Set (False)"=TRUE, "State_In (Wait)"="Wait"}, "State_Machine_Class in"=w523) -> ("error out"=w520:errorcluster, "State_Machine_Class out"=w521:refnum<class "DIO.lvclass">)  [unwired: 6 in, 1 out]
      }
      frame "Wait" {
        n120 = call-dynamic "State_Lock_Unlock.vi"("error in (no error)"=w527, "Parameter"=T4 {"Action_Mode (Get)"=enum."Get", "Action_Set (False)"=FALSE, "State_In (Wait)"="Wait"}, "State_Machine_Class in"=w528) -> ("error out"=w525:errorcluster, "State_Machine_Class out"=w526:refnum<class "DIO.lvclass">)  [unwired: 6 in, 1 out]
      }
      frame "Error_Action" {
        n121 = Variant To Data(error in=w532, type=w532, Variant=w531) -> (data=w533:errorcluster, error out=w530:errorcluster)
        n122 = call <vilib>:"Simple Error Handler.vi"("error in (no error)"=w533) -> ()  [unwired: 4 in, 5 out]
      }
      frame "Stop" {
        n123 = call-dynamic "State_Release.vi"("error in (no error)"=w542, "State_Machine_Class in"=w543) -> ("error out"=w540:errorcluster, "State_Machine_Class out"=w541:refnum<class "DIO.lvclass">)  [unwired: 8 in]
        n124 = call-dynamic "State_Lock_Unlock.vi"("error in (no error)"=w540, "Parameter"=T4 {"Action_Mode (Get)"=enum."Set", "Action_Set (False)"=TRUE, "State_In (Wait)"="Wait"}, "State_Machine_Class in"=w541) -> ("error out"=w537:errorcluster, "State_Machine_Class out"=w539:refnum<class "DIO.lvclass">)  [unwired: 6 in, 1 out]
        n125 = property on="Action Manager" class="Enum (strict)"(error in=w537, "Blinking"=TRUE) -> (error out=w536:errorcluster)  [unwired: 1 in, 1 out]
        n126 = One Button Dialog(message="All State is Locking !\nPlease Unlock With Action Manager to Release . . .") -> ()  [unwired: 1 in, 1 out]
      }
      frame "Exit" {
        n127 = call-dynamic "State_Release.vi"("error in (no error)"=w546, "State_Machine_Class in"=w547) -> ("error out"=w544:errorcluster, "State_Machine_Class out"=w545:refnum<class "DIO.lvclass">)  [unwired: 8 in]
      }
    }
    n128 = case shown="\"Init\"" w142 {
      tunnel: w167 -> [_ _ _ _ _ _ _ _ w412 _ _ w425 _ _]
      tunnel: w166 -> [w360 w362 w370 w372 w377 w386 w399 w406 w410 w417 w422 w424 w434 w438]
      tunnel: w165 -> [w359 w361 w369 w371 w376 w385 w398 w405 w409 w416 w421 w426 w433 w437]
      tunnel: [w357 w362 w366 w372 w375 w382 w397 w404 w410 w415 w420 w424 w429 w436] -> w160
      tunnel: [w356 w361 w365 w371 w374 w381 w396 w403 w408 w414 w419 w423 w428 w435] -> w159
      tunnel: w107 -> [w358 _ _ _ _ _ _ _ _ _ _ _ _ _]
      frame "Idle", Default {
        n129 = call-dynamic "State_Verify.vi"("error in (no error)"=w359, "State(Idle)"=w358, "State_Machine_Class in"=w360) -> ("error out"=w356:errorcluster, "Active"=→"Data_Logging":bool, "State_Machine_Class out"=w357:refnum<class "Data_Logging.lvclass">)  [unwired: 6 in]
      }
      frame "State_Interval" {
        # "Files Monitering or Cirtical Task Handling Here"
      }
      frame "Init" {
        n130 = call-dynamic "State_Interval.vi"("error in (no error)"=w369, "Parameter"=T5 {"Delay(s)"=15.0, "State (Interval_Delay)"="Interval_Delay"}, "State_Machine_Class in"=w370) -> ("error out"=w364:errorcluster, "State_Machine_Class out"=w367:refnum<class "Data_Logging.lvclass">)  [unwired: 6 in, 1 out]
        n131 = call-dynamic "State_Lock_Unlock.vi"("error in (no error)"=w364, "Parameter"=T4 {"Action_Mode (Get)"=enum."Set", "Action_Set (False)"=TRUE, "State_In (Wait)"="Wait"}, "State_Machine_Class in"=w367) -> ("error out"=w365:errorcluster, "State_Machine_Class out"=w366:refnum<class "Data_Logging.lvclass">)  [unwired: 6 in, 1 out]
      }
      frame "Data_Logging" {
        # "Save Data Files Here"
      }
      frame "Set_Interval" {
        n132 = call-dynamic "State_Interval.vi"("error in (no error)"=w376, "Parameter"=T5 {"Delay(s)"=15.0, "State (Interval_Delay)"="Interval_Delay"}, "State_Machine_Class in"=w377) -> ("error out"=w374:errorcluster, "State_Machine_Class out"=w375:refnum<class "Data_Logging.lvclass">)  [unwired: 6 in, 1 out]
      }
      frame "Interval_Delay" {
        n133 = call-dynamic "State_Interval.vi"("error in (no error)"=w385, "Parameter"=T5 {"Delay(s)"=0.0, "State (Interval_Delay)"="Interval_Delay"}, "State_Machine_Class in"=w386) -> ("error out"=w383:errorcluster, "Elapsed Time(s)"=w380:dbl, "State_Machine_Class out"=w384:refnum<class "Data_Logging.lvclass">)  [unwired: 6 in]
        n134 = local write "Data_Logging_Elapsed Time(s)"(w380) -> ()
        n135 = Less Or Equal To 0?(x=w380) -> (x <= 0?=w379:bool)
        n136 = local write "Data_Logging_Time_Act"(w379) -> ()
        n137 = case shown="True" w379 {
          tunnel: w384 -> [w388 w394]
          tunnel: w383 -> [w387 w393]
          tunnel: [w388 w392] -> w382
          tunnel: [w387 w391] -> w381
          frame False {
          }
          frame True {
            n138 = call-dynamic "State_LIFO.vi"("error in (no error)"=w393, "State_Interval(Enable)"=FALSE, "State Machine"=T2 {"Command"="Set_Interval", "Data"=variant} ("State"), "State_Machine_Class in"=w394) -> ("error out"=w391:errorcluster, "State_Machine_Class out"=w392:refnum<class "Data_Logging.lvclass">)  [unwired: 6 in]
          }
        }
      }
      frame "Set_Time_Out" {
        n139 = call-dynamic "State_Time_Out.vi"("error in (no error)"=w398, "Parameter"=T3 {"Enable(True)"=TRUE, "Time Out_State Name"="Get_Time_Out", "Time Target (1s)"=30.0, "Time Out_Reply Message_State"="Interval_Delay"}, "State_Machine_Class in"=w399) -> ("error out"=w396:errorcluster, "State_Machine_Class out"=w397:refnum<class "Data_Logging.lvclass">)  [unwired: 5 in, 2 out]
      }
      frame "Get_Time_Out" {
        # "Messege_Confirm"
        n140 = call-dynamic "State_Time_Out.vi"("error in (no error)"=w405, "Parameter"=T3 {"Enable(True)"=TRUE, "Time Out_State Name"="Get_Time_Out", "Time Target (1s)"=0.0, "Time Out_Reply Message_State"="Messege_Confirm"}, "State_Machine_Class in"=w406) -> ("error out"=w403:errorcluster, "Remaining Time (s)"=→"Data_Logging_Elapsed Time(s)":dbl, "Timeout"=→"Data_Logging_Time_Act":bool, "State_Machine_Class out"=w404:refnum<class "Data_Logging.lvclass">)  [unwired: 5 in]
      }
      frame "Messege_Confirm" {
        n141 = Variant To Data(error in=w409, type="", Variant=w412) -> (data=w407:string, error out=w408:errorcluster)
        n142 = One Button Dialog(message=w407) -> ()  [unwired: 1 in, 1 out]
      }
      frame "Set_Wait" {
        n143 = call-dynamic "State_Lock_Unlock.vi"("error in (no error)"=w416, "Parameter"=T4 {"Action_Mode (Get)"=enum."Set", "Action_Set (False)"=TRUE, "State_In (Wait)"="Wait"}, "State_Machine_Class in"=w417) -> ("error out"=w414:errorcluster, "State_Machine_Class out"=w415:refnum<class "Data_Logging.lvclass">)  [unwired: 6 in, 1 out]
      }
      frame "Wait" {
        n144 = call-dynamic "State_Lock_Unlock.vi"("error in (no error)"=w421, "Parameter"=T4 {"Action_Mode (Get)"=enum."Get", "Action_Set (False)"=TRUE, "State_In (Wait)"="Wait"}, "State_Machine_Class in"=w422) -> ("error out"=w419:errorcluster, "State_Machine_Class out"=w420:refnum<class "Data_Logging.lvclass">)  [unwired: 6 in, 1 out]
      }
      frame "Error_Action" {
        n145 = Variant To Data(error in=w426, type=w426, Variant=w425) -> (data=w427:errorcluster, error out=w423:errorcluster)
        n146 = call <vilib>:"Simple Error Handler.vi"("error in (no error)"=w427) -> ()  [unwired: 4 in, 5 out]
      }
      frame "Stop" {
        n147 = call-dynamic "State_Release.vi"("error in (no error)"=w433, "State_Machine_Class in"=w434) -> ("error out"=w431:errorcluster, "State_Machine_Class out"=w432:refnum<class "Data_Logging.lvclass">)  [unwired: 8 in]
        n148 = call-dynamic "State_Lock_Unlock.vi"("error in (no error)"=w431, "Parameter"=T4 {"Action_Mode (Get)"=enum."Set", "Action_Set (False)"=TRUE, "State_In (Wait)"="Wait"}, "State_Machine_Class in"=w432) -> ("error out"=w428:errorcluster, "State_Machine_Class out"=w429:refnum<class "Data_Logging.lvclass">)  [unwired: 6 in, 1 out]
      }
      frame "Exit" {
        n149 = call-dynamic "State_Release.vi"("error in (no error)"=w437, "State_Machine_Class in"=w438) -> ("error out"=w435:errorcluster, "State_Machine_Class out"=w436:refnum<class "Data_Logging.lvclass">)  [unwired: 8 in]
      }
    }
    n150 = case shown="\"Init\"" w120 {
      tunnel: w126 -> [_ _ _ _ _ _ _ w328 _ _ w342 _ _]
      tunnel: w90 -> [w278 w280 w288 w293 w294 w315 w322 w326 w333 w338 w340 w350 w354]
      tunnel: w127 -> [w277 w279 w287 w292 w302 w314 w321 w325 w332 w337 w341 w349 w353]
      tunnel: [w275 w280 w282 w291 w299 w313 w320 w326 w331 w336 w340 w345 w352] -> w128
      tunnel: [w274 w279 w281 w290 w298 w312 w319 w324 w330 w335 w339 w344 w351] -> w129
      tunnel: w106 -> [w276 _ _ _ _ _ _ _ _ _ _ _ _]
      frame "Idle", Default {
        n151 = call-dynamic "State_Verify.vi"("error in (no error)"=w277, "State(Idle)"=w276, "State_Machine_Class in"=w278) -> ("error out"=w274:errorcluster, "Active"=→"Common":bool, "State_Machine_Class out"=w275:refnum<class "Common_State.lvclass">)  [unwired: 6 in]
      }
      frame "State_Interval" {
        # "Cirtical Task Handling Here"
      }
      frame "Init" {
        n152 = call-dynamic "State_Interval.vi"("error in (no error)"=w287, "Parameter"=T5 {"Delay(s)"=15.0, "State (Interval_Delay)"="Interval_Delay"}, "State_Machine_Class in"=w288) -> ("error out"=w284:errorcluster, "State_Machine_Class out"=w285:refnum<class "Common_State.lvclass">)  [unwired: 6 in, 1 out]
        n153 = call-dynamic "State_Lock_Unlock.vi"("error in (no error)"=w284, "Parameter"=T4 {"Action_Mode (Get)"=enum."Set", "Action_Set (False)"=TRUE, "State_In (Wait)"="Wait"}, "State_Machine_Class in"=w285) -> ("error out"=w281:errorcluster, "State_Machine_Class out"=w282:refnum<class "Common_State.lvclass">)  [unwired: 6 in, 1 out]
      }
      frame "Set_Interval" {
        n154 = call-dynamic "State_Interval.vi"("error in (no error)"=w292, "Parameter"=T5 {"Delay(s)"=15.0, "State (Interval_Delay)"="Interval_Delay"}, "State_Machine_Class in"=w293) -> ("error out"=w290:errorcluster, "State_Machine_Class out"=w291:refnum<class "Common_State.lvclass">)  [unwired: 6 in, 1 out]
      }
      frame "Interval_Delay" {
        n155 = call-dynamic "State_Interval.vi"("error in (no error)"=w302, "Parameter"=T5 {"Delay(s)"=5.0, "State (Interval_Delay)"="Interval_Delay"}, "State_Machine_Class in"=w294) -> ("error out"=w300:errorcluster, "Elapsed Time(s)"=w297:dbl, "State_Machine_Class out"=w301:refnum<class "Common_State.lvclass">)  [unwired: 6 in]
        n156 = local write "Common_Elapsed Time(s)"(w297) -> ()
        n157 = Less Or Equal To 0?(x=w297) -> (x <= 0?=w296:bool)
        n158 = local write "Common_Time_Act"(w296) -> ()
        n159 = case shown="True" w296 {
          tunnel: w301 -> [w304 w310]
          tunnel: w300 -> [w303 w309]
          tunnel: [w304 w308] -> w299
          tunnel: [w303 w307] -> w298
          frame False {
          }
          frame True {
            n160 = call-dynamic "State_LIFO.vi"("error in (no error)"=w309, "State_Interval(Enable)"=FALSE, "State Machine"=T2 {"Command"="Interval_Delay", "Data"=variant} ("State"), "State_Machine_Class in"=w310) -> ("error out"=w307:errorcluster, "State_Machine_Class out"=w308:refnum<class "Common_State.lvclass">)  [unwired: 6 in]
          }
        }
      }
      frame "Set_Time_Out" {
        n161 = call-dynamic "State_Time_Out.vi"("error in (no error)"=w314, "Parameter"=T3 {"Enable(True)"=TRUE, "Time Out_State Name"="Get_Time_Out", "Time Target (1s)"=30.0, "Time Out_Reply Message_State"="Interval_Delay"}, "State_Machine_Class in"=w315) -> ("error out"=w312:errorcluster, "State_Machine_Class out"=w313:refnum<class "Common_State.lvclass">)  [unwired: 5 in, 2 out]
      }
      frame "Get_Time_Out" {
        # "Messege_Confirm"
        # "Messege_Confirm"
        n162 = call-dynamic "State_Time_Out.vi"("error in (no error)"=w321, "Parameter"=T3 {"Enable(True)"=TRUE, "Time Out_State Name"="Get_Time_Out", "Time Target (1s)"=0.0, "Time Out_Reply Message_State"="Set_Interval"}, "State_Machine_Class in"=w322) -> ("error out"=w319:errorcluster, "Remaining Time (s)"=→"Common_Elapsed Time(s)":dbl, "Timeout"=→"Common_Time_Act":bool, "State_Machine_Class out"=w320:refnum<class "Common_State.lvclass">)  [unwired: 5 in]
      }
      frame "Messege_Confirm" {
        n163 = Variant To Data(error in=w325, type="", Variant=w328) -> (data=w323:string, error out=w324:errorcluster)
        n164 = One Button Dialog(message=w323) -> ()  [unwired: 1 in, 1 out]
      }
      frame "Set_Wait" {
        n165 = call-dynamic "State_Lock_Unlock.vi"("error in (no error)"=w332, "Parameter"=T4 {"Action_Mode (Get)"=enum."Set", "Action_Set (False)"=TRUE, "State_In (Wait)"="Wait"}, "State_Machine_Class in"=w333) -> ("error out"=w330:errorcluster, "State_Machine_Class out"=w331:refnum<class "Common_State.lvclass">)  [unwired: 6 in, 1 out]
      }
      frame "Wait" {
        n166 = call-dynamic "State_Lock_Unlock.vi"("error in (no error)"=w337, "Parameter"=T4 {"Action_Mode (Get)"=enum."Get", "Action_Set (False)"=FALSE, "State_In (Wait)"="Wait"}, "State_Machine_Class in"=w338) -> ("error out"=w335:errorcluster, "State_Machine_Class out"=w336:refnum<class "Common_State.lvclass">)  [unwired: 6 in, 1 out]
      }
      frame "Error_Action" {
        n167 = Variant To Data(error in=w341, type=w341, Variant=w342) -> (data=w343:errorcluster, error out=w339:errorcluster)
        n168 = call <vilib>:"Simple Error Handler.vi"("error in (no error)"=w343) -> ()  [unwired: 4 in, 5 out]
      }
      frame "Stop" {
        n169 = call-dynamic "State_Release.vi"("error in (no error)"=w349, "State_Machine_Class in"=w350) -> ("error out"=w347:errorcluster, "State_Machine_Class out"=w348:refnum<class "Common_State.lvclass">)  [unwired: 8 in]
        n170 = call-dynamic "State_Lock_Unlock.vi"("error in (no error)"=w347, "Parameter"=T4 {"Action_Mode (Get)"=enum."Set", "Action_Set (False)"=TRUE, "State_In (Wait)"="Wait"}, "State_Machine_Class in"=w348) -> ("error out"=w344:errorcluster, "State_Machine_Class out"=w345:refnum<class "Common_State.lvclass">)  [unwired: 6 in, 1 out]
      }
      frame "Exit" {
        n171 = call-dynamic "State_Release.vi"("error in (no error)"=w353, "State_Machine_Class in"=w354) -> ("error out"=w351:errorcluster, "State_Machine_Class out"=w352:refnum<class "Common_State.lvclass">)  [unwired: 8 in]
      }
    }
    n172 = case shown="\"Init\"" w103 {
      tunnel: w100 -> [_ _ _ _ _ _ _ w246 _ _ w260 _ _]
      tunnel: w99 -> [w197 w199 w203 w212 w221 w233 w240 w244 w251 w256 w258 w268 w272]
      tunnel: w98 -> [w196 w198 w201 w211 w220 w232 w239 w243 w250 w255 w259 w267 w271]
      tunnel: [w194 w199 w207 w210 w217 w231 w238 w244 w249 w254 w258 w263 w270] -> w96
      tunnel: [w193 w198 w206 w209 w216 w230 w237 w242 w248 w253 w257 w262 w269] -> w94
      tunnel: w95 -> [w195 _ _ _ _ _ _ _ _ _ _ _ _]
      frame "Idle", Default {
        n173 = call-dynamic "State_Verify.vi"("error in (no error)"=w196, "State(Idle)"=w195, "State_Machine_Class in"=w197) -> ("error out"=w193:errorcluster, "Active"=→"Base Class":bool, "State_Machine_Class out"=w194:refnum<class "Hyper_State_Machine.lvclass">)  [unwired: 6 in]
      }
      frame "State_Interval" {
        # "Cirtical Task Handling Here"
      }
      frame "Init" {
        n174 = call-dynamic "State_Time_Out.vi"("error in (no error)"=w201, "Parameter"=T3 {"Enable(True)"=TRUE, "Time Out_State Name"="Get_Time_Out", "Time Target (1s)"=10.0, "Time Out_Reply Message_State"="Get_Time_Out"}, "State_Machine_Class in"=w203) -> ("error out"=w200:errorcluster, "State_Machine_Class out"=w202:refnum<class "Hyper_State_Machine.lvclass">)  [unwired: 5 in, 2 out]
        n175 = call-dynamic "State_Lock_Unlock.vi"("error in (no error)"=w200, "Parameter"=T4 {"Action_Mode (Get)"=enum."Set", "Action_Set (False)"=TRUE, "State_In (Wait)"="Wait"}, "State_Machine_Class in"=w202) -> ("error out"=w206:errorcluster, "State_Machine_Class out"=w207:refnum<class "Hyper_State_Machine.lvclass">)  [unwired: 6 in, 1 out]
      }
      frame "Set_Interval" {
        n176 = call-dynamic "State_Interval.vi"("error in (no error)"=w211, "Parameter"=T5 {"Delay(s)"=15.0, "State (Interval_Delay)"="Interval_Delay"}, "State_Machine_Class in"=w212) -> ("error out"=w209:errorcluster, "State_Machine_Class out"=w210:refnum<class "Hyper_State_Machine.lvclass">)  [unwired: 6 in, 1 out]
      }
      frame "Interval_Delay" {
        n177 = call-dynamic "State_Interval.vi"("error in (no error)"=w220, "Parameter"=T5 {"Delay(s)"=0.0, "State (Interval_Delay)"="Interval_Delay"}, "State_Machine_Class in"=w221) -> ("error out"=w218:errorcluster, "Elapsed Time(s)"=w215:dbl, "State_Machine_Class out"=w219:refnum<class "Hyper_State_Machine.lvclass">)  [unwired: 6 in]
        n178 = local write "Base Class_Elapsed Time(s)"(w215) -> ()
        n179 = Less Or Equal To 0?(x=w215) -> (x <= 0?=w214:bool)
        n180 = local write "Base Class_Time_Act"(w214) -> ()
        n181 = case shown="True" w214 {
          tunnel: w219 -> [w223 w228]
          tunnel: w218 -> [w222 w227]
          tunnel: [w223 w226] -> w217
          tunnel: [w222 w225] -> w216
          frame False {
          }
          frame True {
            n182 = call-dynamic "State_LIFO.vi"("error in (no error)"=w227, "State Machine"=T2 {"Command"="Set_Interval", "Data"=variant} ("State"), "State_Machine_Class in"=w228) -> ("error out"=w225:errorcluster, "State_Machine_Class out"=w226:refnum<class "Hyper_State_Machine.lvclass">)  [unwired: 7 in]
          }
        }
      }
      frame "Set_Time_Out" {
        n183 = call-dynamic "State_Time_Out.vi"("error in (no error)"=w232, "Parameter"=T3 {"Enable(True)"=TRUE, "Time Out_State Name"="Get_Time_Out", "Time Target (1s)"=30.0, "Time Out_Reply Message_State"="Interval_Delay"}, "State_Machine_Class in"=w233) -> ("error out"=w230:errorcluster, "State_Machine_Class out"=w231:refnum<class "Hyper_State_Machine.lvclass">)  [unwired: 5 in, 2 out]
      }
      frame "Get_Time_Out" {
        # "Messege_Confirm"
        n184 = call-dynamic "State_Time_Out.vi"("error in (no error)"=w239, "Parameter"=T3 {"Enable(True)"=TRUE, "Time Out_State Name"="Get_Time_Out", "Time Target (1s)"=5.0, "Time Out_Reply Message_State"="Get_Time_Out"}, "State_Machine_Class in"=w240) -> ("error out"=w237:errorcluster, "Remaining Time (s)"=→"Base Class_Elapsed Time(s)":dbl, "Timeout"=→"Base Class_Time_Act":bool, "State_Machine_Class out"=w238:refnum<class "Hyper_State_Machine.lvclass">)  [unwired: 5 in]
      }
      frame "Messege_Confirm" {
        n185 = Variant To Data(error in=w243, type="", Variant=w246) -> (data=w241:string, error out=w242:errorcluster)
        n186 = One Button Dialog(message=w241) -> ()  [unwired: 1 in, 1 out]
      }
      frame "Set_Wait" {
        n187 = call-dynamic "State_Lock_Unlock.vi"("error in (no error)"=w250, "Parameter"=T4 {"Action_Mode (Get)"=enum."Set", "Action_Set (False)"=TRUE, "State_In (Wait)"="Wait"}, "State_Machine_Class in"=w251) -> ("error out"=w248:errorcluster, "State_Machine_Class out"=w249:refnum<class "Hyper_State_Machine.lvclass">)  [unwired: 6 in, 1 out]
      }
      frame "Wait" {
        n188 = call-dynamic "State_Lock_Unlock.vi"("error in (no error)"=w255, "Parameter"=T4 {"Action_Mode (Get)"=enum."Get", "Action_Set (False)"=FALSE, "State_In (Wait)"="Wait"}, "State_Machine_Class in"=w256) -> ("error out"=w253:errorcluster, "State_Machine_Class out"=w254:refnum<class "Hyper_State_Machine.lvclass">)  [unwired: 6 in, 1 out]
      }
      frame "Error_Action" {
        n189 = Variant To Data(error in=w259, type=w259, Variant=w260) -> (data=w261:errorcluster, error out=w257:errorcluster)
        n190 = call <vilib>:"Simple Error Handler.vi"("error in (no error)"=w261) -> ()  [unwired: 4 in, 5 out]
      }
      frame "Stop" {
        n191 = call-dynamic "State_Release.vi"("error in (no error)"=w267, "State_Machine_Class in"=w268) -> ("error out"=w265:errorcluster, "State_Machine_Class out"=w266:refnum<class "Hyper_State_Machine.lvclass">)  [unwired: 8 in]
        n192 = call-dynamic "State_Lock_Unlock.vi"("error in (no error)"=w265, "Parameter"=T4 {"Action_Mode (Get)"=enum."Set", "Action_Set (False)"=TRUE, "State_In (Wait)"="Wait"}, "State_Machine_Class in"=w266) -> ("error out"=w262:errorcluster, "State_Machine_Class out"=w263:refnum<class "Hyper_State_Machine.lvclass">)  [unwired: 6 in, 1 out]
      }
      frame "Exit" {
        n193 = call-dynamic "State_Release.vi"("error in (no error)"=w271, "State_Machine_Class in"=w272) -> ("error out"=w269:errorcluster, "State_Machine_Class out"=w270:refnum<class "Hyper_State_Machine.lvclass">)  [unwired: 8 in]
      }
    }
    n194 = case "Commander" shown="\"Init\"" w191 {
      tunnel: w190 -> [_ _ _ _ _ _ _ w818 w826 _ _ _ w852 _ _]
      tunnel: w188 -> [w753 w755 w762 w780 w790 w805 w812 w816 w822 w836 w844 w848 w853 w860 w865]
      tunnel: w187 -> [w751 w754 w761 w779 w789 w804 w811 w815 w825 _ w843 w847 w849 w859 w864]
      tunnel: [w750 w755 w764 w778 w785 w803 w810 w816 w822 w836 w842 w846 w853 w856 w863] -> w112
      tunnel: [w749 w754 w763 w777 w784 w802 w809 w814 w821 w835 w841 w845 w850 w855 w862] -> w186
      tunnel: [_ _ _ _ _ _ _ _ _ _ _ _ _ _ TRUE] -> w189
      tunnel: w111 -> [w752 _ _ _ w781 _ _ _ _ _ _ _ _ _ _]
      tunnel: w177 -> [_ _ _ _ _ _ _ _ _ _ _ _ _ _ _]
      tunnel: w77 -> [_ _ _ _ _ _ _ _ _ w833 _ _ _ _ _]
      tunnel: w76 -> [_ _ _ _ _ _ _ _ _ w832 _ _ _ _ _]
      tunnel: w75 -> [_ _ _ _ _ _ _ _ _ w831 _ _ _ _ _]
      tunnel: w74 -> [_ _ _ _ _ _ _ _ _ w830 _ _ _ _ _]
      tunnel: w73 -> [_ _ _ _ _ _ _ _ _ w829 _ _ _ _ _]
      tunnel: w72 -> [_ _ _ _ _ _ _ _ _ w828 _ _ _ _ _]
      frame "Idle", Default {
        n195 = call-dynamic "State_Verify.vi"("error in (no error)"=w751, "State(Idle)"=w752, "State_Machine_Class in"=w753) -> ("error out"=w749:errorcluster, "Active"=→"Commander":bool, "State_Machine_Class out"=w750:refnum<class "Commander.lvclass">)  [unwired: 6 in]
      }
      frame "State_Interval" {
      }
      frame "Init" {
        # "Test Using Static Delay (2s) + SetInterval (3s) = 5 sec"
        n196 = call-dynamic "Product_Activate.vi"("error in (no error)"=w761, "Activate Code"="Activate_Code(Blank for 30 min Trial)", "Commander in"=w762) -> ("error out"=w759:errorcluster, "Activate"=→"Activate":bool, "Product ID"=→"Product ID":string, "Commander out"=w760:refnum<class "Commander.lvclass">)  [unwired: 5 in]
        n197 = disable-structure shown="Enabled" {
          disable-tunnel: [w769 w774] -> w764
          disable-tunnel: [w768 w773] -> w763
          disable-tunnel: w760 -> [w766 w775]
          disable-tunnel: w759 -> [w765 w772]
          frame Disabled {
            n198 = call-dynamic "State_Interval.vi"("error in (no error)"=w765, "Parameter"=T5 {"Delay(s)"=5.0, "State (Interval_Delay)"="Interval_Delay"}, "State_Machine_Class in"=w766) -> ("error out"=w768:errorcluster, "State_Machine_Class out"=w769:refnum<class "Commander.lvclass">)  [unwired: 6 in, 1 out]
          }
          frame Enabled {
            n199 = Build Array(T2 {"Command"="Interval_Delay", "Data"=variant} ("State")) -> (w770:T2[])
            n200 = call-dynamic "State_FIFO.vi"("error in (no error)"=w772, "State Machine[]"=w770, "State_Machine_Class in"=w775) -> ("error out"=w773:errorcluster, "State_Machine_Class out"=w774:refnum<class "Commander.lvclass">)  [unwired: 7 in]
          }
        }
      }
      frame "Set_Interval" {
        n201 = call-dynamic "State_Interval.vi"("error in (no error)"=w779, "Parameter"=T5 {"Delay(s)"=3.0, "State (Interval_Delay)"="Interval_Delay"}, "State_Machine_Class in"=w780) -> ("error out"=w777:errorcluster, "State_Machine_Class out"=w778:refnum<class "Commander.lvclass">)  [unwired: 6 in, 1 out]
      }
      frame "Interval_Delay" {
        n202 = call-dynamic "State_Interval.vi"("error in (no error)"=w789, "Parameter"=T5 {"Delay(s)"=2.0, "State (Interval_Delay)"="Interval_Delay"}, "State_Machine_Class in"=w790) -> ("error out"=w786:errorcluster, "Elapsed Time(s)"=w783:dbl, "State_Machine_Class out"=w787:refnum<class "Commander.lvclass">)  [unwired: 6 in]
        "Commander_Elapsed Time(s)" <- w783
        n203 = Less Or Equal To 0?(x=w783) -> (x <= 0?=w788:bool)
        n204 = local write "State1_Time_Act"(w788) -> ()
        n205 = case shown="True" w788 {
          tunnel: w787 -> [w792 w800]
          tunnel: w786 -> [w791 w799]
          tunnel: [w792 w798] -> w785
          tunnel: [w791 w797] -> w784
          tunnel: w781 -> [_ w796]
          frame False {
          }
          frame True {
            n206 = Build Array(w796, T2 {"Command"="Set_Interval", "Data"=variant} ("State"), T2 {"Command"="Member_Release", "Data"=variant} ("State")) -> (w793:T2[])
            n207 = call-dynamic "State_FIFO.vi"("error in (no error)"=w799, "State Machine[]"=w793, "State_Machine_Class in"=w800) -> ("error out"=w797:errorcluster, "State_Machine_Class out"=w798:refnum<class "Commander.lvclass">)  [unwired: 7 in]
          }
        }
      }
      frame "Set_Time_Out" {
        n208 = call-dynamic "State_Time_Out.vi"("error in (no error)"=w804, "Parameter"=T3 {"Enable(True)"=TRUE, "Time Out_State Name"="Get_Time_Out", "Time Target (1s)"=30.0, "Time Out_Reply Message_State"="Messege_Confirm"}, "State_Machine_Class in"=w805) -> ("error out"=w802:errorcluster, "State_Machine_Class out"=w803:refnum<class "Commander.lvclass">)  [unwired: 5 in, 2 out]
      }
      frame "Get_Time_Out" {
        n209 = call-dynamic "State_Time_Out.vi"("error in (no error)"=w811, "Parameter"=T3 {"Enable(True)"=TRUE, "Time Out_State Name"="Get_Time_Out", "Time Target (1s)"=0.0, "Time Out_Reply Message_State"="Messege_Confirm"}, "State_Machine_Class in"=w812) -> ("error out"=w809:errorcluster, "Remaining Time (s)"=w808:dbl, "Timeout"=→"State1_Time_Act":bool, "State_Machine_Class out"=w810:refnum<class "Commander.lvclass">)  [unwired: 5 in]
        n210 = local write "Commander_Elapsed Time(s)"(w808) -> ()
      }
      frame "Messege_Confirm" {
        n211 = Variant To Data(error in=w815, type="", Variant=w818) -> (data=w813:string, error out=w814:errorcluster)
        n212 = One Button Dialog(message=w813) -> ()  [unwired: 1 in, 1 out]
      }
      frame "Dynamics_Release" {
        n213 = Variant To Data(error in=w825, type=refnum<class "Hyper_State_Machine.lvclass"> refnum ("SSW_Hyper_State_Machine.lvlibp:Hyper_State_Machine.lvclass"), Variant=w826) -> (data=w824:refnum<class "Hyper_State_Machine.lvclass">, error out=w823:errorcluster)
        n214 = call-dynamic "State_Lock_Unlock.vi"("error in (no error)"=w823, "Parameter"=T4 {"Action_Mode (Get)"=enum."Set", "Action_Set (False)"=FALSE, "State_In (Wait)"="Wait"}, "State_Machine_Class in"=w824) -> ("error out"=w821:errorcluster)  [unwired: 6 in, 2 out]
      }
      frame "Member_Release" {
        n215 = Build Array(w833, w832, w831, w830, w829, w828) -> (w827:refnum<class "Hyper_State_Machine.lvclass">[])
        n216 = for {
          tunnel: [w839] -> w835
          tunnel: T4 {"Action_Mode (Get)"=enum."Set", "Action_Set (False)"=FALSE, "State_In (Wait)"="Wait"} ("Parameter") -> [w838]
          tunnel: w827 -> [w837] mode=indexing
          n217 = call-dynamic "State_Lock_Unlock.vi"("Parameter"=w838, "State_Machine_Class in"=w837) -> ("error out"=w839:errorcluster)  [unwired: 7 in, 2 out]
        }
      }
      frame "Set_Wait" {
        n218 = call-dynamic "State_Lock_Unlock.vi"("error in (no error)"=w843, "Parameter"=T4 {"Action_Mode (Get)"=enum."Set", "Action_Set (False)"=TRUE, "State_In (Wait)"="Wait"}, "State_Machine_Class in"=w844) -> ("error out"=w841:errorcluster, "State_Machine_Class out"=w842:refnum<class "Commander.lvclass">)  [unwired: 6 in, 1 out]
      }
      frame "Wait" {
        n219 = call-dynamic "State_Lock_Unlock.vi"("error in (no error)"=w847, "State_Machine_Class in"=w848) -> ("error out"=w845:errorcluster, "State_Machine_Class out"=w846:refnum<class "Commander.lvclass">)  [unwired: 7 in, 1 out]
      }
      frame "Error_Action" {
        n220 = Variant To Data(error in=w849, type=w849, Variant=w852) -> (data=w851:errorcluster, error out=w850:errorcluster)
        n221 = call <vilib>:"Simple Error Handler.vi"("error in (no error)"=w851) -> ()  [unwired: 4 in, 5 out]
      }
      frame "Stop" {
        n222 = call-dynamic "State_Release.vi"("error in (no error)"=w859, "State_Machine_Class in"=w860) -> ("error out"=w857:errorcluster, "State_Machine_Class out"=w858:refnum<class "Commander.lvclass">)  [unwired: 8 in]
        n223 = call-dynamic "State_Lock_Unlock.vi"("error in (no error)"=w857, "Parameter"=T4 {"Action_Mode (Get)"=enum."Set", "Action_Set (False)"=TRUE, "State_In (Wait)"="Wait"}, "State_Machine_Class in"=w858) -> ("error out"=w855:errorcluster, "State_Machine_Class out"=w856:refnum<class "Commander.lvclass">)  [unwired: 6 in, 1 out]
      }
      frame "Exit" {
        n224 = call-dynamic "State_Release.vi"("error in (no error)"=w864, "State_Machine_Class in"=w865) -> ("error out"=w862:errorcluster, "State_Machine_Class out"=w863:refnum<class "Commander.lvclass">)  [unwired: 8 in]
      }
    }
    n225 = local read "Heart_Rate"() -> (w88:bool)
    n226 = Or(x=w189, y=w174) -> (x .or. y?=w175:bool)
    n227 = Not(x=w88) -> (.not. x?=→"Heart_Rate":bool)
    n228 = call <vilib>:"High Resolution Polling Wait.vi"("seconds to wait"="System_Wait_Time") -> ()  [unwired: 10 in, 1 out]
    n229 = call-dynamic "State_Error_Handling.vi"("error in (no error)"=w170, "Reply_State_Name"=w91, "Handling_State(State_Acquisition)"=w110, "State_Machine_Class in"=w171) -> ("error out"=w178:errorcluster, "State_Machine_Class out"=w179:refnum<class "Image_Acquisition.lvclass">)  [unwired: 6 in]
    n230 = call-dynamic "State_Error_Handling.vi"("error in (no error)"=w155, "Reply_State_Name"=w91, "Handling_State(State_Acquisition)"=w109, "State_Machine_Class in"=w158) -> ("error out"=w149:errorcluster, "State_Machine_Class out"=w154:refnum<class "Motion_Control.lvclass">)  [unwired: 6 in]
    n231 = call-dynamic "State_Error_Handling.vi"("error in (no error)"=w161, "Reply_State_Name"=w91, "Handling_State(State_Acquisition)"=w108, "State_Machine_Class in"=w162) -> ("error out"=w148:errorcluster, "State_Machine_Class out"=w153:refnum<class "DIO.lvclass">)  [unwired: 6 in]
    n232 = call-dynamic "State_Error_Handling.vi"("error in (no error)"=w159, "Reply_State_Name"=w91, "Handling_State(State_Acquisition)"=w107, "State_Machine_Class in"=w160) -> ("error out"=w146:errorcluster, "State_Machine_Class out"=w147:refnum<class "Data_Logging.lvclass">)  [unwired: 6 in]
    n233 = call-dynamic "State_Error_Handling.vi"("error in (no error)"=w129, "Reply_State_Name"=w91, "Handling_State(State_Acquisition)"=w106, "State_Machine_Class in"=w128) -> ("error out"=w123:errorcluster, "State_Machine_Class out"=w124:refnum<class "Common_State.lvclass">)  [unwired: 6 in]
    n234 = call-dynamic "State_Error_Handling.vi"("error in (no error)"=w94, "Reply_State_Name"=w91, "Handling_State(State_Acquisition)"=w95, "State_Machine_Class in"=w96) -> ("error out"=w93:errorcluster, "State_Machine_Class out"=w92:refnum<class "Hyper_State_Machine.lvclass">)  [unwired: 6 in]
    n235 = call-dynamic "State_Error_Handling.vi"("error in (no error)"=w186, "Reply_State_Name"=w91, "Handling_State(State_Acquisition)"=w111, "State_Machine_Class in"=w112) -> ("error out"=w185:errorcluster, "State_Machine_Class out"=w184:refnum<class "Commander.lvclass">)  [unwired: 6 in]
  }
  n236 = while {
    tunnel: w7 -> [w873]
    tunnel: w6 -> [w872]
    tunnel: w5 -> [w871]
    tunnel: w4 -> [w870]
    tunnel: w3 -> [w869]
    tunnel: w2 -> [w868]
    tunnel: w1 -> [w866]
    stop <- w867 stop-if-true
    n237 = event shown="[0] Timeout" {
      selector: _ -> [_ _ _]
      dyn-events: _ -> [_ _ _]
      timeout: _ -> [_ _ _]
      tunnel: w873 -> [_ w884 w918]
      tunnel: w872 -> [_ w883 _]
      tunnel: w871 -> [_ w882 _]
      tunnel: w870 -> [_ w881 _]
      tunnel: w869 -> [_ w880 _]
      tunnel: w868 -> [_ w879 _]
      tunnel: [_ _ TRUE] -> w867
      tunnel: w866 -> [_ w877 _]
      event Timeout {
        n238 = event-data() -> ()  [unwired: 1 in, 3 out]
      }
      event "Action Manager": Value Change {
        n239 = event-data() -> ("NewVal"=w878:T1)  [unwired: 1 in]
        n240 = Build Array(w884, w883, w882, w881, w880, w879, w877) -> (w885:refnum<class "Hyper_State_Machine.lvclass">[])
        n241 = case shown="\"Init\"" w878 {
          tunnel: w885 -> [_ w890 w898 w905 w912]
          tunnel: [w886 w888 w897 w904 w910] -> w876
          tunnel: errorcluster {"status"=FALSE, "code"=0, "source"=""} ("error out") -> [w886 w889 w896 w903 w911]
          frame "No Action", Default {
          }
          frame "Init" {
            n242 = for {
              tunnel: w890 -> [w895] mode=indexing
              shift-right: [w892] -> w888
              shift-left: w889 -> [w894]
              tunnel: T2 {"Command"="Init", "Data"=variant} ("State") -> [w891]
              n243 = call-dynamic "State_LIFO.vi"("error in (no error)"=w894, "State_Interval(Enable)"=FALSE, "State Machine"=w891, "State_Machine_Class in"=w895) -> ("error out"=w892:errorcluster)  [unwired: 6 in, 1 out]
            }
          }
          frame "Lock" {
            n244 = for {
              tunnel: w898 -> [w902] mode=indexing
              shift-right: [w900] -> w897
              shift-left: w896 -> [w899]
              n245 = call-dynamic "State_Lock_Unlock.vi"("error in (no error)"=w899, "Parameter"=T4 {"Action_Mode (Get)"=enum."Set", "Action_Set (False)"=TRUE, "State_In (Wait)"="Wait"}, "State_Machine_Class in"=w902) -> ("error out"=w900:errorcluster)  [unwired: 6 in, 2 out]
            }
          }
          frame "Unlock" {
            n246 = for {
              tunnel: w905 -> [w909] mode=indexing
              shift-right: [w907] -> w904
              shift-left: w903 -> [w906]
              n247 = call-dynamic "State_Lock_Unlock.vi"("error in (no error)"=w906, "Parameter"=T4 {"Action_Mode (Get)"=enum."Set", "Action_Set (False)"=FALSE, "State_In (Wait)"="Wait"}, "State_Machine_Class in"=w909) -> ("error out"=w907:errorcluster)  [unwired: 6 in, 2 out]
            }
          }
          frame "Release" {
            n248 = for {
              tunnel: w912 -> [w915] mode=indexing
              shift-right: [w913] -> w910
              shift-left: w911 -> [w914]
              n249 = call-dynamic "State_Release.vi"("error in (no error)"=w914, "State_Machine_Class in"=w915) -> ("error out"=w913:errorcluster)  [unwired: 8 in, 1 out]
            }
          }
        }
        n250 = property on="Action Manager" class="Enum (strict)"(error in=w876, "Blinking"=FALSE) -> ()  [unwired: 1 in, 2 out]
      }
      event "Stop": Value Change {
        n251 = event-data() -> ()  [unwired: 1 in, 6 out]
        n252 = call-dynamic "State_LIFO.vi"("State_Interval(Enable)"=FALSE, "State Machine"=T2 {"Command"="Exit", "Data"=variant} ("State"), "State_Machine_Class in"=w918) -> ()  [unwired: 7 in, 2 out]
      }
    }
  }
  n253 = call-dynamic "State_Destroy.vi"("error in (no error)"=w59, "State_Machine_Class in"=w60) -> ("error out"=w57:errorcluster)  [unwired: 8 in, 1 out]
  n254 = call-dynamic "State_Destroy.vi"("error in (no error)"=w48, "State_Machine_Class in"=w51) -> ("error out"=w42:errorcluster)  [unwired: 8 in, 1 out]
  n255 = call-dynamic "State_Destroy.vi"("error in (no error)"=w46, "State_Machine_Class in"=w50) -> ("error out"=w41:errorcluster)  [unwired: 8 in, 1 out]
  n256 = call-dynamic "State_Destroy.vi"("error in (no error)"=w44, "State_Machine_Class in"=w45) -> ("error out"=w40:errorcluster)  [unwired: 8 in, 1 out]
  n257 = call-dynamic "State_Destroy.vi"("error in (no error)"=w36, "State_Machine_Class in"=w37) -> ("error out"=w35:errorcluster)  [unwired: 8 in, 1 out]
  n258 = call-dynamic "State_Destroy.vi"("error in (no error)"=w31, "State_Machine_Class in"=w30) -> ("error out"=w29:errorcluster)  [unwired: 8 in, 1 out]
  n259 = call-dynamic "State_Destroy.vi"("error in (no error)"=w63, "State_Machine_Class in"=w62) -> ("error out"=w58:errorcluster)  [unwired: 8 in, 1 out]
  n260 = Merge Errors(w58, w57, w42, w41, w40, w35, w29) -> (w56:errorcluster)
  n261 = call <vilib>:"Simple Error Handler.vi"("error in (no error)"=w56) -> ()  [unwired: 4 in, 5 out]
